vi "Main.vi"() -> ()   [LabVIEW 2017]
uses:
  type defs/action buttons.ctl
  type defs/mode buttons.ctl
  <vilib>/vision/Pattern Matching.llb/IMAQ GM Match Report.ctl
  type defs/states.ctl
  type defs/data.ctl
  <vilib>/vision/Image Controls.llb/IMAQ Image.ctl
  <vilib>/myRIO/Common/Instrument Driver Framework/myRIO v1.0/Encoder/typedefs/Encoder Signal Mode.ctl
  <vilib>/myRIO/Instrument Drivers/Onboard IO/PWM/typedefs/PWM Reference.ctl
  <vilib>/myRIO/Common/Instrument Driver Framework/Utilities/typedefs/myRIO Generic Hardware Reference.ctl
  <vilib>/myRIO/Common/Instrument Driver Framework/Utilities/typedefs/Hardware Version Enum.ctl
  <vilib>/myRIO/Common/Instrument Driver Framework/Utilities/typedefs/myRIO v1.0 Reference.ctl
  <vilib>/myRIO/Common/Instrument Driver Framework/Utilities/typedefs/Generic FPGA Reference.ctl
  <vilib>/myRIO/Common/Instrument Driver Framework/myRIO v1.0/PWM/typedefs/PWM Channels Enum.ctl
  <vilib>/myRIO/Instrument Drivers/Onboard IO/PWM/typedefs/PWM Configuration.ctl
  <vilib>/userdefined/High Color/nirio_resource_hc.ctl
  <vilib>/myRIO/Instrument Drivers/Onboard IO/DIO/typedefs/DIO Reference.ctl
  <vilib>/myRIO/Common/Instrument Driver Framework/myRIO v1.0/DIO/typedefs/DIO Channels List.ctl
  <vilib>/myRIO/Common/Instrument Driver Framework/myRIO v1.0/DIO/typedefs/DIO Channels Enum.ctl
  type defs/task.ctl
  <vilib>/myRIO/Common/Instrument Driver Framework/Utilities/vis/Is FPGA Ref Available.vi
  <vilib>/myRIO/Common/Instrument Driver Framework/myRIO v1.0/PWM/vis/myRIO v1.1 Open PWM.vi
  <vilib>/myRIO/Common/Instrument Driver Framework/myRIO v1.0/DIO/vis/myRIO v1.1 Open DIO.vi
  <vilib>/myRIO/Instrument Drivers/Onboard IO/DIO/vis/Write.vi
  <vilib>/myRIO/Common/Instrument Driver Framework/Utilities/vis/Validate Channels.vi
  <vilib>/myRIO/Common/Instrument Driver Framework/myRIO v1.0/PWM/vis/myRIO v1.0 Reserve PWM.vi
  <vilib>/myRIO/Common/Instrument Driver Framework/myRIO v1.0/DIO/vis/myRIO v1.0 Reserve DIO.vi
  <vilib>/myRIO/Common/Instrument Driver Framework/myRIO v1.0/Encoder/vis/myRIO v1.0 Close Encoder.vi
  <vilib>/myRIO/Common/Instrument Driver Framework/myRIO v1.0/PWM/vis/myRIO v1.0 Close PWM.vi
  <vilib>/myRIO/Common/Instrument Driver Framework/myRIO v1.0/UART/vis/myRIO v1.0 Close UART.vi
  <vilib>/myRIO/Common/Instrument Driver Framework/myRIO v1.0/PWM/vis/myRIO v1.0 Build MUX Configuration PWM.vi
  <vilib>/myRIO/Common/Instrument Driver Framework/myRIO v1.0/Resource Manager/vis/myRIO v1.0 Reserve Channel List.vi
  <vilib>/myRIO/Common/Instrument Driver Framework/myRIO v1.0/DIO/vis/myRIO v1.0 Build MUX Configuration DIO.vi
  <vilib>/myRIO/Common/Instrument Driver Framework/myRIO v1.0/Encoder/vis/myRIO v1.0 Unreserve Encoder.vi
  <vilib>/myRIO/Common/Instrument Driver Framework/myRIO v1.0/PWM/vis/myRIO v1.0 Unreserve PWM.vi
  <vilib>/myRIO/Common/Instrument Driver Framework/myRIO v1.0/Resource Manager/vis/myRIO v1.0 Create Configuration List.vi
  <vilib>/myRIO/Common/Instrument Driver Framework/myRIO v1.0/Resource Manager/vis/myRIO v1.0 Reserve Channel.vi
  <vilib>/myRIO/Common/Instrument Driver Framework/myRIO v1.0/Resource Manager/vis/myRIO v1.0 Unreserve Channel.vi
  <vilib>/myRIO/Common/Instrument Driver Framework/myRIO v1.0/Encoder/vis/myRIO v1.0 Build MUX Configuration Encoder.vi
  <vilib>/myRIO/Common/Instrument Driver Framework/myRIO v1.0/Resource Manager/vis/myRIO v1.0 Unreserve Channel List.vi
  <vilib>/myRIO/Common/Instrument Driver Framework/myRIO v1.0/Resource Manager/vis/myRIO v1.0 Build Mutex Name.vi
  <vilib>/Utility/VariantDataType/GetNumericInfo.vi
  <vilib>/Utility/error.llb/Error Cluster From Error Code.vi
  <vilib>/myRIO/Common/Instrument Driver Framework/myRIO v1.0/myRIO v1.1 Open.vi
  <vilib>/myRIO/Common/Instrument Driver Framework/Utilities/vis/IO Manager.vi
  <vilib>/myRIO/Common/Instrument Driver Framework/Utilities/vis/Configuration Manager.vi
  <vilib>/myRIO/Common/Instrument Driver Framework/myRIO v1.0/Resource Manager/vis/myRIO v1.0 Configure IO.vi
  <vilib>/myRIO/Common/Instrument Driver Framework/myRIO v1.0/myRIO v1.0 Close.vi
  <vilib>/myRIO/Common/Instrument Driver Framework/myRIO v1.0/Encoder/vis/myRIO v1.0 Reset Encoder.vi
  <vilib>/myRIO/Common/Instrument Driver Framework/myRIO v1.0/PWM/vis/myRIO v1.0 Write PWM.vi
  <vilib>/myRIO/Common/Instrument Driver Framework/myRIO v1.0/Encoder/vis/myRIO v1.0 Read Encoder.vi
  <vilib>/myRIO/Common/Instrument Driver Framework/myRIO v1.0/DIO/vis/myRIO v1.0 Write DIO.vi
  <vilib>/myRIO/Common/Instrument Driver Framework/myRIO v1.0/DIO/vis/myRIO v1.0 Read DIO.vi
  <vilib>/myRIO/Common/Instrument Driver Framework/myRIO v1.0/PWM/vis/myRIO v1.0 Shutdown PWM.vi
  <vilib>/myRIO/Common/Instrument Driver Framework/myRIO v1.0/Encoder/vis/myRIO v1.0 Shutdown Encoder.vi
  <vilib>/myRIO/Common/Instrument Driver Framework/Utilities/vis/FPGA Ref Manager.vi
  <vilib>/myRIO/Common/Instrument Driver Framework/myRIO v1.0/myRIO v1.0 Reset FPGA.vi
  <vilib>/myRIO/Common/Instrument Driver Framework/myRIO v1.0/IRQ/vis/myRIO v1.0 IRQ Info FGV.vi
  <vilib>/myRIO/Common/Instrument Driver Framework/myRIO v1.0/IRQ/vis/myRIO v1.0 Timer IRQ Info FGV.vi
  <vilib>/myRIO/Common/Instrument Driver Framework/myRIO v1.0/IRQ/vis/myRIO v1.0 ISR Agent.vi
  <vilib>/myRIO/Instrument Drivers/Onboard IO/I2C/typedefs/I2C Reference.ctl
  <vilib>/myRIO/Common/Instrument Driver Framework/myRIO v1.0/I2C/typedefs/I2C Channels Enum.ctl
  <vilib>/myRIO/Instrument Drivers/Onboard IO/I2C/typedefs/I2C Configuration.ctl
  <vilib>/myRIO/Instrument Drivers/Onboard IO/I2C/typedefs/I2C Transfer Rate.ctl
  <vilib>/myRIO/Express VI/Onboard IO/PWM/PWM Express VI.xnode
  <vilib>/myRIO/Instrument Drivers/Onboard IO/PWM/vis/myRIO PWM Open.xnode
  <vilib>/myRIO/Express VI/Onboard IO/DO/DO Express VI.xnode
  <vilib>/myRIO/Instrument Drivers/Onboard IO/DIO/vis/myRIO DIO Open.xnode
  <vilib>/myRIO/Express VI/Onboard Devices/LED/LED Express VI.xnode
  <vilib>/myRIO/Express VI/Onboard Devices/Button/Button Express VI.xnode
  <vilib>/myRIO/Instrument Drivers/Onboard IO/DIO/DIO.lvlib
  <vilib>/myRIO/Instrument Drivers/Onboard IO/PWM/PWM.lvlib
  <vilib>/myRIO/Instrument Drivers/Utilities/Utilities.lvlib
  <vilib>/vision/NI_Vision_Development_Module.lvlib
  <vilib>/myRIO/Instrument Drivers/Onboard IO/I2C/I2C.lvlib
  <vilib>/myRIO/Instrument Drivers/Onboard IO/I2C/vis/myRIO I2C Open.xnode
  <vilib>/myRIO/Common/Instrument Driver Framework/myRIO v1.0/I2C/vis/myRIO v1.1 Open I2C.vi
  <vilib>/myRIO/Instrument Drivers/Onboard IO/Encoder/Encoder.lvlib
panel:
  in  "Def PWM":dbl=0.5
  out "CurState":T1(ring)
  out "Found Right Ball":bool=TRUE
  out "FT_G_enc":i32[](array[numeric])
  out "FT_M_enc":i32[](array[numeric])
  out "FT_Right_enc":i32[](array[numeric])
  out "FT_Left_enc":i32[](array[numeric])
  out "FT_Angles":dbl[](array[numeric])
  out "Dots of States":i32[][](array[numeric])
  in  "States in total":i32
  in  "(auto) States":T2(ring)
  out "G_enc":i32[](array[numeric])
  out "M_enc":i32[](array[numeric])
  out "Right_enc":i32[](array[numeric])
  out "Left_enc":i32[](array[numeric])
  out "Angles":dbl[](array[numeric])
  in  "Dots in total":i32
  in  "CurDot":T3(ring)
  out "(auto) balls counter":i32
  out "distance to the side":u32
  out "value Z 2":ext
  out "value Z":ext
  in  ",ctl num":i32
  in  ".Task":enum16{"Def", "<mod>[P]+tnl ", "(auto)"}(ring)
  out "Pattern classes":i32[](array[numeric])
  in  "5":i32
  in  "4":i32
  in  "3":i32
  in  "1":i32
  in  "2":i32
  out "5b":bool
  out "4b":bool
  out "3b":bool
  out "2b":bool
  out "1b":bool
  out "Color classes":i32[](array[numeric])
  in  "Next step":bool
  in  "ball = pattern?":bool
  out "error out":errorcluster
  in  "Tab Control":enum32{"Motors", "Ball", "Pattern", "Camera"}(tab)
  in  "Left+":bool
  in  "Left-":bool
  in  "Right+":bool
  in  "Right-":bool
  in  "G-":bool
  in  "G+":bool
  in  "M+":bool
  in  "M-":bool
  in  "M_PWM":dbl=0.5
  in  "L_PWM":dbl=0.5
  in  "R_PWM":dbl=0.5
  in  "Reset M_enc":bool
  out "M_enc_value":i32
  in  "Reset G_enc":bool
  out "G_enc_value":i32
  in  "G_PWM":dbl=0.5
  in  "M_UB_Align":i32=-800
  in  "G_UB_Align":i32
  in  "M_UB_grab":i32=-800
  in  "G_UB_grab":i32=-500
  in  "Manip state":enum16{"Align", "Grab", "Release"}(ring)
  in  "Reset L_enc":bool
  out "L_enc_value":i32
  in  "Reset R_enc":bool
  out "R_enc_value":i32
  in  "Balls to remember":i32
  out "Circles Calibrated (Shape Detection 1)":T4(array[cluster]) {"Position"."Y" format="%.2f"; "Position"."X" format="%.2f"}
  out "Number of Matches (Shape Detection 1)":i32
  out "Color":i32
  in  "Align X - t, Y - f":bool
  out "CircleRadius":dbl
  in  "defX":dbl=360.0
  in  "RangeY":dbl=30.0
  in  "defY":dbl=380.0
  out "X is in range":bool
  out "Y is in range":bool
  out "curX":dbl
  out "curY":dbl
  out "1y1 (circle)":i32
  out "1x1 (circle)":i32
  out "1x0 (circle)":i32
  out "1y0 (circle)":i32
  in  "divider (circle)":dbl=1.0
  in  "ROI Descriptor COLOR":T5={"Global Rectangle"=[86, 71, 180, 164], "Contours"=[{"ID"=enum."External", "Type"=3, "Coordinates"=[86, 71, 180, 164]}]} {"Contours"."Type" items=["No Selection", "Point", "Line", "Rectangle", "Oval", "Polygon", "Freehand Region", "Annulus", "Unused2", "Unused3", "Broken Line", "Freehand Line", "Rotated Rectangle"]}
  in  "align accuracy":u32=100
  in  "Ball number":i32=1
  out "ball match":bool
  in  "RangeX":dbl=40.0
  out "Ready to Grab":bool
  in  "Range(p)":sgl=10.0
  in  "defX(p)":sgl=320.0
  out "Pattern":i32
  out "y0":i32
  out "x0":i32
  out "x1":i32
  out "y1":i32
  out "Number of Matches (Geometric Matching 1)":i32
  out "Calibrated Matches (Geometric Matching 1)":T6[](array[typedef]) {"Correlation Score" format="%.2f"; "Target Template Curve Score" format="%.2f"; "Template Target Curve Score" format="%.2f"; "Bounding Box"."y" format="%.2f"; "Bounding Box"."x" format="%.2f"; "Position"."y" format="%.2f"; "Position"."x" format="%.2f"; "Score" format="%.2f"; "Scale" format="%.2f"; "Angle" format="%.2f"; "Occlusion %" format="%.2f"}
  out "Scale":sgl
  in  "divider (pattern)":sgl=1.0
  out "curX(p)":sgl
  out "In Range? (p)":bool
  in  "align accuracy (p)":u32=100
  in  "pattern number":i32=1
  in  "patterns to remember":i32=3
  out "pattern match":bool
  in  "M duty cycle [P]":dbl=533.0 format="%#_13g"
  in  "S duty cycle [P]":dbl=990.0 format="%#_13g"
  in  "S duty cycle [B]":dbl=990.0 format="%#_13g"
  in  "M duty cycle [B]":dbl=533.0 format="%#_13g"
  in  "S duty cycle [F]":dbl=620.0 format="%#_13g"
  in  "M duty cycle [F]":dbl=506.0 format="%#_13g"
  in  "Angle for pattern (degrees)":sgl=90.0 format="%.2f"
  out "rotate":bool=TRUE
  in  "PWM channel (m)":tag="B/PWM2"
  in  "[cur] duty cycle [%] (m)":dbl
  in  "PWM channel (s)":tag="A/PWM2"
  in  "[cur] duty cycle [%] (s)":dbl
  in  "Camera state":enum16{"Fwd", "Pattern", "Ball"}(ring)
  in  "Angle for Align (degrees)":sgl=2.0 format="%.2f"
  in  "mode buttons":T7
  out "image display":T8(plugin-control)
  in  "action buttons":T9
  in  "Stop":bool
  # "Machine\nVision\nApp"
  # "less = slower"
  # "less = slower"
  # "0 - 640x480"
  # "5 - 1280x720"
  # "30 - 320x240"
  # "35 - 800x600"
  # "40 - 176x144"
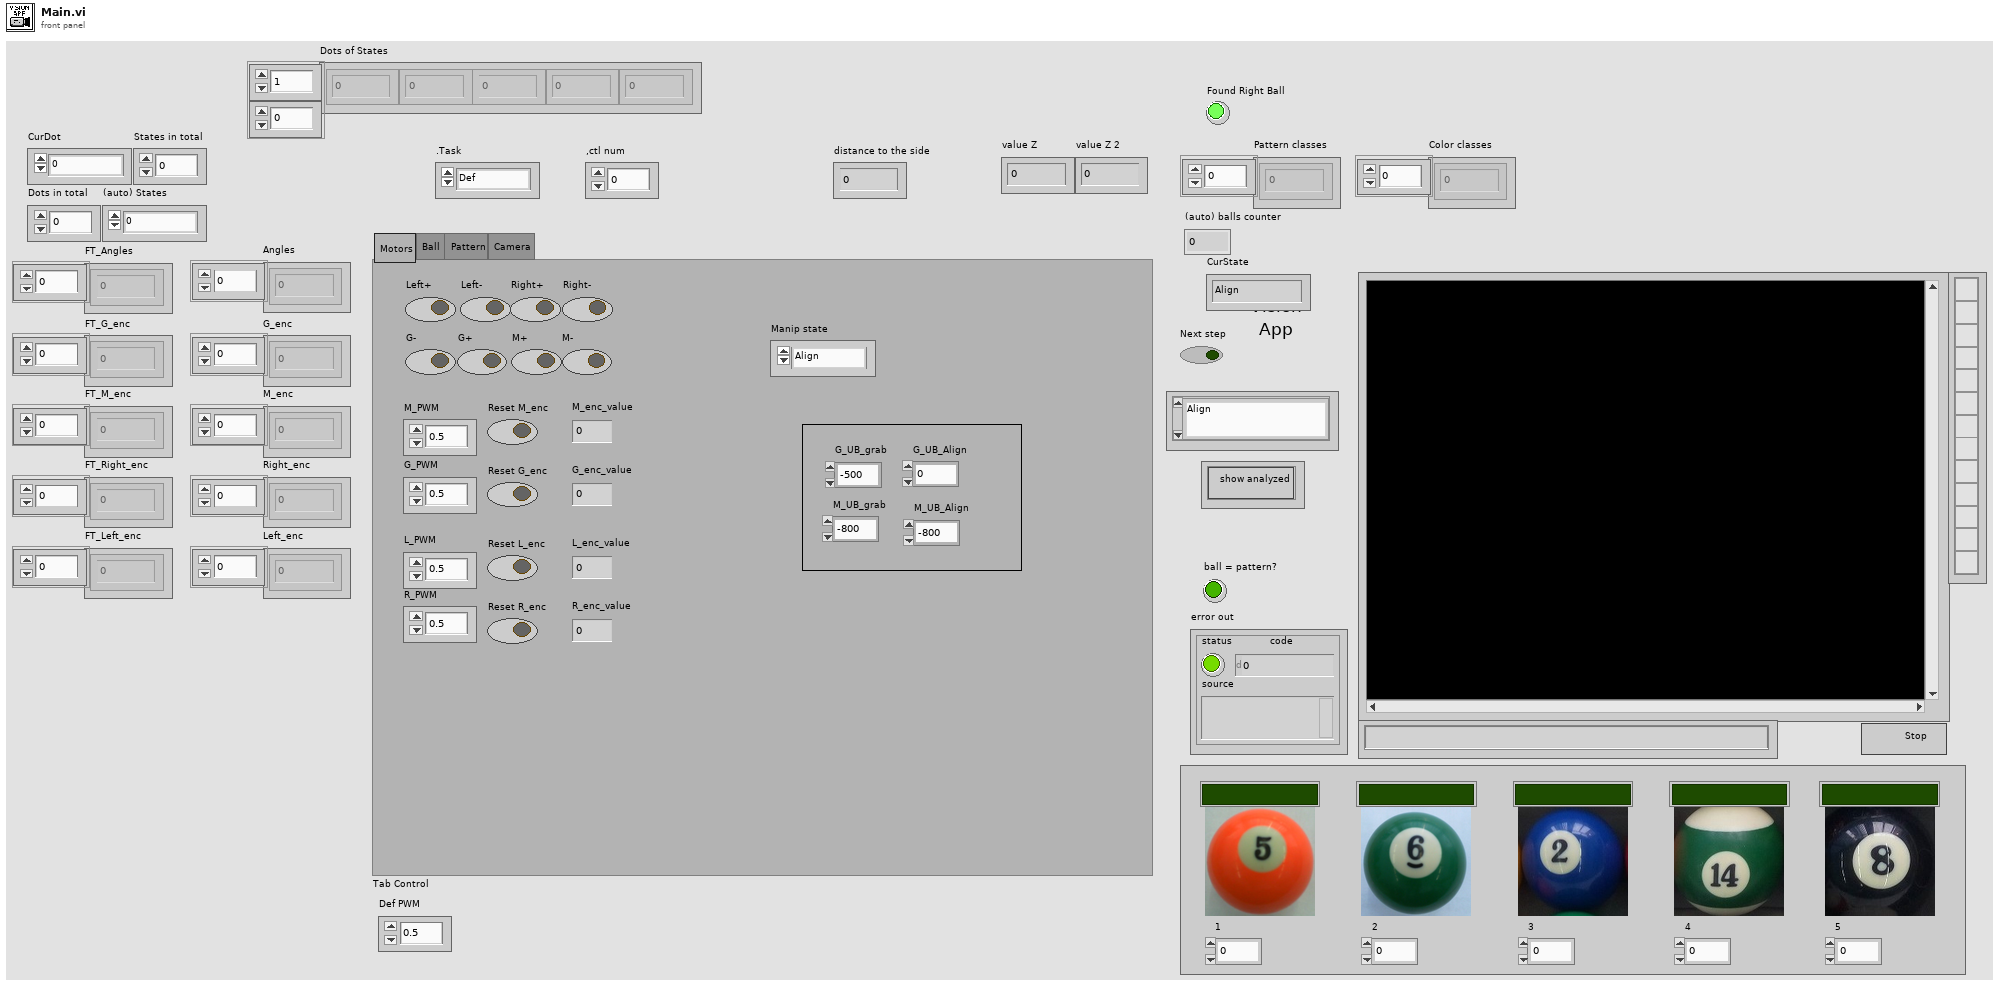
[diagram p1: front panel]
types:
  T1 = enum16{"Align", "1", "2", "3", "4", "5", "6", "7", "8", "9", "10", "11", "12", "13", "(pattern) Align", "Pattern", "(mod) pattern", "<mod>[P] remembering", "<mod>[P] go through tunnel", "<mod>[P] comparing", "(mod) ball", "Ball", "Other", "Clear", "navx", "(auto) Balls Analyze", "(auto) Ball Analyze", "(pattern) Align <loop>", "(ball) Align <loop>", "Joystick control"}
  T2 = enum16{"0", "1", "2", "3", "4", "5", "6", "7", "8", "9", "10"}
  T3 = enum16{"0", "1", "2", "3", "4", "5", "6", "7", "8", "9", "10", "11", "12", "13", "14", "15", "16", "17", "18", "19", "20", "21", "22", "23", "24", "25", "26", "27", "28", "29", "30", "31", "32", "33", "34", "35"}
  T4 = cluster{"Position":cluster{"X":sgl, "Y":sgl}, "Radius":dbl, "Score":dbl}[]
  T5 = cluster{"Global Rectangle":i32[], "Contours":cluster{"ID":enum32{"External", "Internal"}, "Type":u32, "Coordinates":i32[]}[]}
  T6 = typedef "IMAQ GM Match Report.ctl" = cluster{"Position":cluster{"x":sgl, "y":sgl}, "Angle":sgl, "Scale":sgl, "Score":sgl, "Bounding Box":cluster{"x":sgl, "y":sgl}[], "Contrast Reversed":bool, "Occlusion %":sgl, "Template Target Curve Score":sgl, "Target Template Curve Score":sgl, "Correlation Score":sgl}
  T7 = typedef "mode buttons.ctl" = cluster{"show analyzed":bool}
  T8 = typedef "IMAQ Image.ctl" = refnum<image>
  T9 = typedef "action buttons.ctl" = cluster{"State":enum16{"Align", "1", "2", "3", "4", "5", "6", "7", "8", "9", "10", "11", "12", "13", "(pattern) Align", "Pattern", "(mod) pattern", "<mod>[P] remembering", "<mod>[P] go through tunnel", "<mod>[P] comparing", "(mod) ball", "Ball", "Other", "Clear", "navx", "(auto) Balls Analyze", "(auto) Ball Analyze", "(pattern) Align <loop>", "(ball) Align <loop>", "Joystick control"}}
  T10 = typedef "Encoder Signal Mode.ctl" = enum16{"Quadrature phase signal", "Step and direction signal"}
  T11 = typedef "data.ctl" = cluster{"Shape - t, Color - f":bool, "qsm":cluster{"Webcam image ref":T8, "Analyzed image ref":T8, "Stop webcam":bool}, " image ref":T8, "number img":i32, "ROI Descriptor (Image Mask 1)":cluster{"Global Rectangle":i32[], "Contours":cluster{"ID":enum32{"External", "Internal"}, "Type":u32, "Coordinates":i32[]}[]}, "Pattern class":i32, "Color class":i32, "Color classes":i32[], "Pattern classes":i32[]}
  T12 = typedef "states.ctl" = enum16{"(qsm) schedule", "(qsm) initialize", "(qsm) release", "(qsm) clean up", "(qsm) shutdown", "(myRIO) initialize", "(myRIO) clean up", "(myRIO) update ports", "Setup get", "(image) get", "(image) show", "(ball) Shape detection", "(ball) Calc ball indx", "(ball) Calculate ROI", "(ball) Analyze color", "(ball) Align", "(ball) Wait", "(ball) Grab", "(pattern) Find Square", "(pattern) Calculate ROI", "(pattern) Calc pattern indx", "Compare", "(pattern) Analyze pattern", "(pattern) Align", "(pattern) Wait", "(pattern) states control", "navx", "stop motors", "(joystick) Joystick control", "_Timer", "Setup manipulator", "(auto) Count balls", "(auto) Analyze balls", "(auto) Dot Controller", "(auto) Fwd (cm)", "(auto) Turn (angle)", "(auto) Tnl (M2-M2.5)", "Wait for button"}
  T13 = typedef "Encoder.lvlib/Encoder Reference.ctl" = cluster{"myRIO Reference":T14, "Encoder Channels Enum":T18}
  T14 = typedef "myRIO Generic Hardware Reference.ctl" = cluster{"myRIO Model":T15, "myRIO Hardware Reference":T16}
  T15 = typedef "Hardware Version Enum.ctl" = enum16{"Unknown", "myRIO-1900", "myRIO-1950", "roboRIO", "NI ELVIS RIO CM"}
  T16 = typedef "myRIO v1.0 Reference.ctl" = cluster{"Generic FPGA Reference":T17, "Allow multiple opens":bool}
  T17 = typedef "Generic FPGA Reference.ctl" = refnum<k20>
  T18 = typedef "Encoder Channels Enum.ctl" = enum16{"Not Connected", "C/ENC0", "C/ENC1", "A/ENC", "B/ENC", "DIO/ENC0", "DIO/ENC1", "DIO/ENC2", "DIO/ENC3", "DIO/ENC4"}
  T19 = typedef "PWM.lvlib/PWM Reference.ctl" = cluster{"myRIO Reference":T14, "PWM Channels Enum":T20, "PWM Configuration":T21}
  T20 = typedef "PWM Channels Enum.ctl" = enum16{"Not Connected", "C/PWM0", "C/PWM1", "A/PWM0", "A/PWM1", "A/PWM2", "B/PWM0", "B/PWM1", "B/PWM2", "PWM/PWM0", "PWM/PWM1", "PWM/PWM2", "PWM/PWM3", "PWM/PWM4", "PWM/PWM5", "PWM/PWM6", "PWM/PWM7", "PWM/PWM8", "PWM/PWM9"}
  T21 = typedef "PWM.lvlib/PWM Configuration.ctl" = cluster{"Frequency":dbl, "Duty Cycle":dbl}
  T22 = typedef "nirio_resource_hc.ctl" = tag
  T23 = typedef "I2C.lvlib/I2C Reference.ctl" = cluster{"myRIO Reference":T14, "I2C Channels Enum":T24, "I2C Configuration":T25}
  T24 = typedef "I2C Channels Enum.ctl" = enum16{"Not Connected", "A/I2C", "B/I2C", "I2C/I2C"}
  T25 = typedef "I2C.lvlib/I2C Configuration.ctl" = cluster{"I2C Transfer Rate":T26}
  T26 = typedef "I2C.lvlib/I2C Transfer Rate.ctl" = enum16{"Standard mode (100 kbps)", "Fast mode (400 kbps)"}
  T27 = typedef "DIO.lvlib/DIO Reference.ctl" = cluster{"myRIO Reference":T14, "DIO Channels List":T28}
  T28 = typedef "DIO Channels List.ctl" = T29[]
  T29 = typedef "DIO Channels Enum.ctl" = enum16{"Not Connected", "C/DIO0", "C/DIO1", "C/DIO2", "C/DIO3", "C/DIO4", "C/DIO5", "C/DIO6", "C/DIO7", "A/DIO0", "A/DIO1", "A/DIO2", "A/DIO3", "A/DIO4", "A/DIO5", "A/DIO6", "A/DIO7", "A/DIO8", "A/DIO9", "A/DIO10", "A/DIO11", "A/DIO12", "A/DIO13", "A/DIO14", "A/DIO15", "B/DIO0", "B/DIO1", "B/DIO2", "B/DIO3", "B/DIO4", "B/DIO5", "B/DIO6", "B/DIO7", "B/DIO8", "B/DIO9", "B/DIO10", "B/DIO11", "B/DIO12", "B/DIO13", "B/DIO14", "B/DIO15", "LED0", "LED1", "LED2", "LED3", "Button0", "DIO/DIO0", "DIO/DIO1", "DIO/DIO2", "DIO/DIO3", "DIO/DIO4", "DIO/DIO5", "DIO/DIO6", "DIO/DIO7", "DIO/DIO8", "DIO/DIO9", "SPI/CS0", "SPI/CS1", "SPI/CS2", "SPI/CS3", "LED RADIO (Green)", "LED RADIO (Red)", "LED COMM (Green)", "LED COMM (Red)", "LED MODE (Green)", "LED MODE (Red)"}
  T30 = enum16{"Align", "(pattern) Align", "Pattern", "(mod) pattern", "(mod) ball", "Ball", "Other", "Clear", "Joystick control"}
  T31 = enum16{"Align", "(pattern) Align", "Pattern", "(mod) pattern", "<mod>[P] remembering", "<mod>[P] go through tunnel", "<mod>[P] comparing", "(mod) ball", "Ball", "Other", "Clear", "Joystick control"}
  T32 = enum16{"Align", "(pattern) Align", "Pattern", "(mod) pattern", "<mod>[P]+move", "(mod) ball", "Ball", "Other", "Clear", "Joystick control"}
  T33 = typedef "task.ctl" = T12[]
  T34 = typedef "Image Type" = u32
  T35 = cluster{"Position":cluster{"X":sgl, "Y":sgl}, "Radius":dbl, "Score":dbl}
  T36 = cluster{"ID":enum32{"External", "Internal"}, "Type":u32, "Coordinates":i32[]}[]
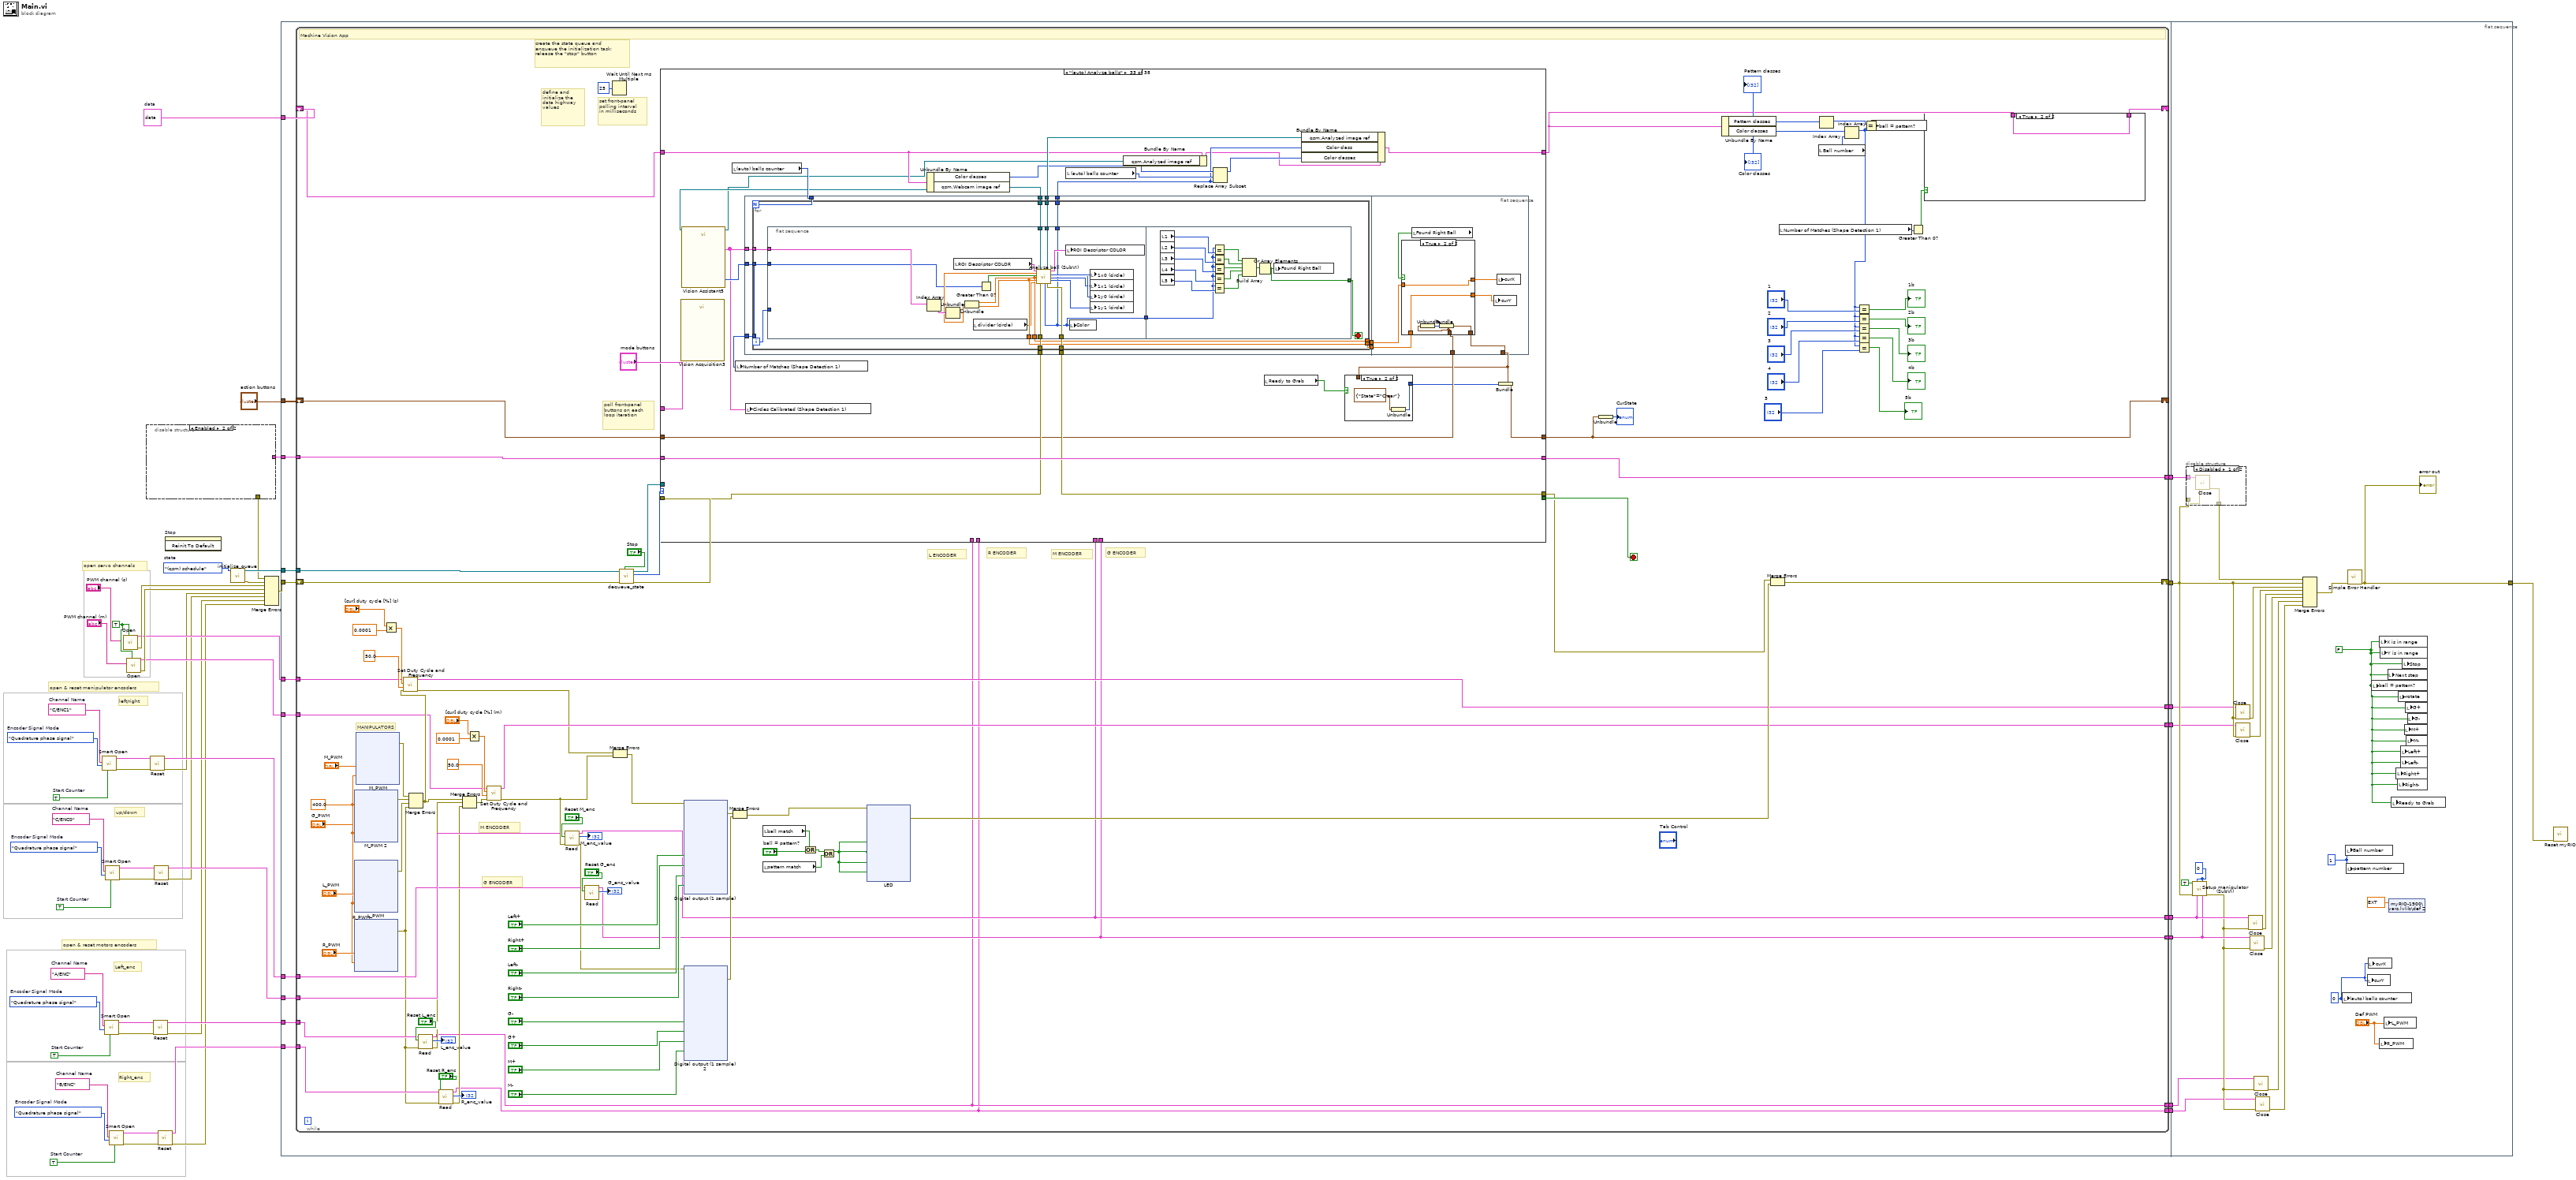
[diagram p0: block diagram]
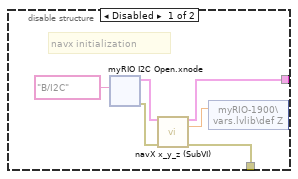
[diagram p2: hidden frame]
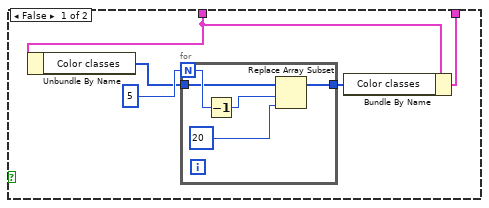
[diagram p3: hidden frame]
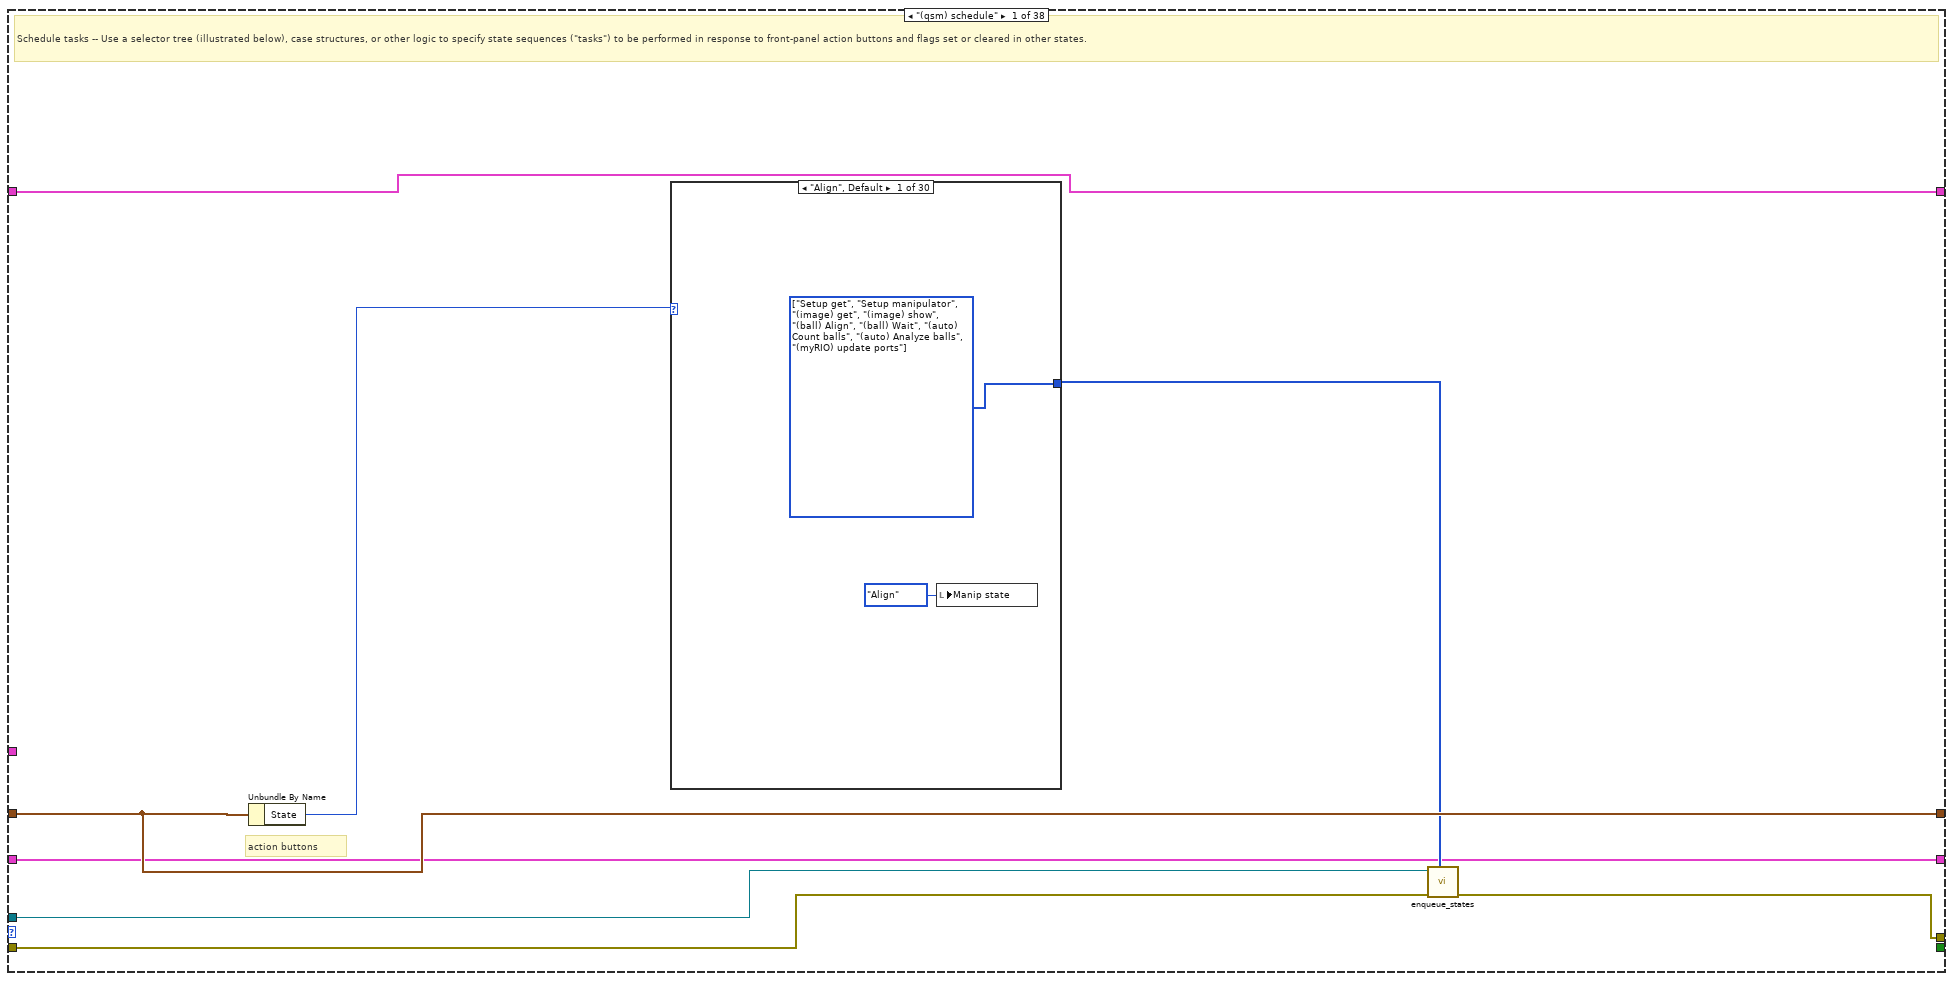
[diagram p4: hidden frame]
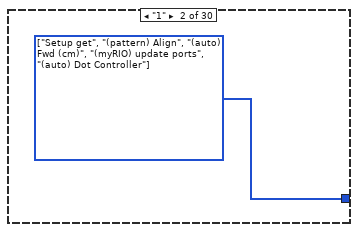
[diagram p5: hidden frame]
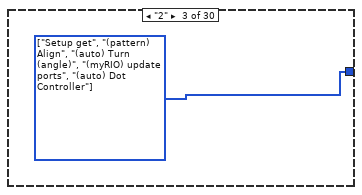
[diagram p6: hidden frame]
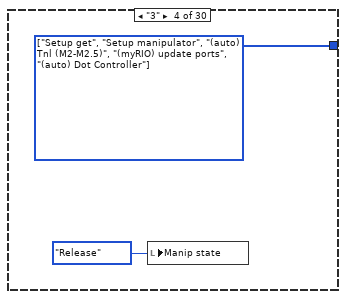
[diagram p7: hidden frame]
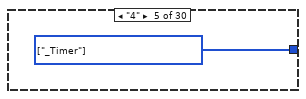
[diagram p8: hidden frame]
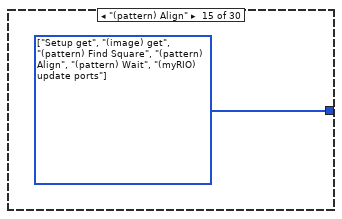
[diagram p18: hidden frame]
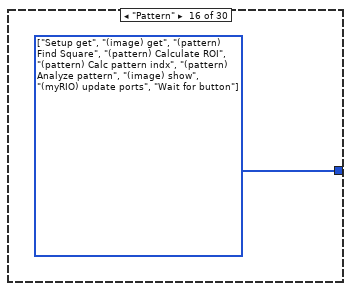
[diagram p19: hidden frame]
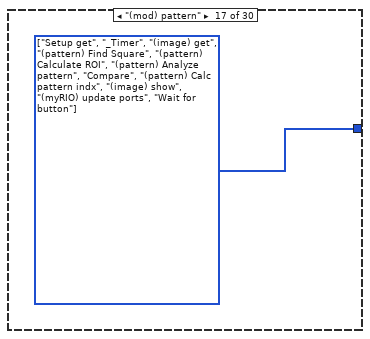
[diagram p20: hidden frame]
diagram:
  w8 = TRUE  # Start Counter
  w7 = TRUE  # Start Counter
  w11 = Encoder_Signal_Mode."Quadrature phase signal"  # Encoder Signal Mode
  w12 = tag "B/ENC"  # Channel Name
  w15 = Encoder_Signal_Mode."Quadrature phase signal"  # Encoder Signal Mode
  w16 = tag "A/ENC"  # Channel Name
  w24 = TRUE  # Start Counter
  w25 = Encoder_Signal_Mode."Quadrature phase signal"  # Encoder Signal Mode
  w26 = tag "C/ENC1"  # Channel Name
  w30 = TRUE  # Start Counter
  w31 = Encoder_Signal_Mode."Quadrature phase signal"  # Encoder Signal Mode
  w32 = tag "C/ENC0"  # Channel Name
  w39 = TRUE ("Allow multiple opens?")
  w36 = T11 {"Shape - t, Color - f"=FALSE, "qsm"={"Webcam image ref"=refnum, "Analyzed image ref"=refnum, "Stop webcam"=FALSE}, " image ref"=refnum, "number img"=0, "ROI Descriptor (Image Mask 1)"={"Global Rectangle"=[109, 72, 345, 284], "Contours"=[{"ID"=enum."External", "Type"=3, "Coordinates"=[109, 72, 345, 284]}]}, "Pattern class"=0, "Color class"=0, "Color classes"=[], "Pattern classes"=[]}  # data
  w47 = states."(qsm) schedule"  # state
  # "open & reset motors encoders"
  # "Right_enc"
  # "Left_enc"
  # "left/right"
  # "up/down"
  # "open servo channels"
  # "open & reset manipulator encoders"
  n1 = call <vilib>:"Smart Open.vi"("Start Counter"=w24, "Encoder Signal Mode"=w25, "Channel Name"=w26) -> ("error out"=w22:errorcluster, "Encoder Ref Out"=w23:T13)  [unwired: 7 in]
  n2 = call <vilib>:"Smart Open.vi"("Start Counter"=w7, "Encoder Signal Mode"=w15, "Channel Name"=w16) -> ("error out"=w13:errorcluster, "Encoder Ref Out"=w14:T13)  [unwired: 7 in]
  n3 = call <vilib>:"Smart Open.vi"("Start Counter"=w30, "Encoder Signal Mode"=w31, "Channel Name"=w32) -> ("error out"=w28:errorcluster, "Encoder Ref Out"=w29:T13)  [unwired: 7 in]
  n4 = call <vilib>:"Smart Open.vi"("Start Counter"=w8, "Encoder Signal Mode"=w11, "Channel Name"=w12) -> ("error out"=w9:errorcluster, "Encoder Ref Out"=w10:T13)  [unwired: 7 in]
  n5 = call <vilib>:"Open.vi"("Allow multiple opens?"=w39, "Channel Name"="PWM channel (s)") -> ("error out"=w45:errorcluster, "PWM Ref Out"=w43:T19)  [unwired: 8 in]
  n6 = call <vilib>:"Open.vi"("Allow multiple opens?"=w39, "Channel Name"="PWM channel (m)") -> ("error out"=w44:errorcluster, "PWM Ref Out"=w42:T19)  [unwired: 8 in]
  n7 = disable-structure shown="Enabled" {
    disable-tunnel: [w56 _] -> w34
    disable-tunnel: [w54 _] -> w33
    frame Disabled {
      # "navx initialization"
      n8 = xnode "myRIO I2C Open.xnode"("Channel Name"=tag "B/I2C") -> ("error out"=w53:errorcluster, "I2C Ref Out"=w55:T23)  [unwired: 2 in]
      n9 = call "navX x_y_z (SubVI).vi"("I2C Ref Out in"=w55, "error in (no error)"=w53) -> ("I2C Ref Out out"=w54:T23, "value Z"=w57:ext, "error out"=w56:errorcluster)  [unwired: 9 in, 2 out]
      n10 = shared-variable "myRIO-1900\\vars.lvlib\\def Z"(w57) -> ()  [unwired: 1 in, 1 out]
    }
    frame Enabled {
    }
  }
  n11 = call <vilib>:"Reset.vi"("error in (no error)"=w22, "Encoder Ref In"=w23) -> ("error out"=w17:errorcluster, "Encoder Ref Out"=w21:T13)  [unwired: 8 in]
  n12 = call <vilib>:"Reset.vi"("error in (no error)"=w13, "Encoder Ref In"=w14) -> ("error out"=w4:errorcluster, "Encoder Ref Out"=w6:T13)  [unwired: 8 in]
  n13 = call <vilib>:"Reset.vi"("error in (no error)"=w28, "Encoder Ref In"=w29) -> ("error out"=w18:errorcluster, "Encoder Ref Out"=w27:T13)  [unwired: 8 in]
  n14 = call <vilib>:"Reset.vi"("error in (no error)"=w9, "Encoder Ref In"=w10) -> ("error out"=w3:errorcluster, "Encoder Ref Out"=w5:T13)  [unwired: 8 in]
  n15 = invoke on="Stop" class="Bool (strict)" method="Reinit To Default"() -> ()  [unwired: 3 in, 3 out]
  n16 = call "initialize_queue.vi"("state"=w47) -> ("error out"=w48:errorcluster, "queue out"=w49:refnum<queue>)  [unwired: 9 in]
  n17 = Merge Errors(w34, w48, w45, w44, w17, w18, w4, w3) -> (w46:errorcluster)
  n18 = flat-sequence {
    tunnel: [w93] -> w51
    tunnel: "action buttons" -> [w92]
    tunnel: w46 -> [w90]
    tunnel: w49 -> [w91]
    tunnel: w36 -> [w89]
    tunnel: w43 -> [w88]
    tunnel: w42 -> [w87]
    tunnel: [w86] -> w41
    tunnel: [w85] -> w40
    tunnel: w33 -> [w84]
    tunnel: [w83] -> w35
    tunnel: w27 -> [w82]
    tunnel: w21 -> [w81]
    tunnel: [w80] -> w20
    tunnel: [w79] -> w19
    tunnel: w6 -> [w78]
    tunnel: w5 -> [w77]
    tunnel: [w76] -> w2
    tunnel: [w75] -> w1
    tunnel: [w1391] -> w52
    tunnel: w51 -> [w1381]
    tunnel: w41 -> [w1379]
    tunnel: w40 -> [w1378]
    tunnel: w35 -> [w1386]
    tunnel: w20 -> [w1376]
    tunnel: w19 -> [w1377]
    tunnel: w2 -> [w1372]
    tunnel: w1 -> [w1373]
    frame #0 {
      n19 = while {
        shift-right: [w186] -> w93
        shift-left: w90 -> [w191]
        shift-right: [w167] -> _
        shift-left: w89 -> [w94]
        shift-right: [w97] -> _
        shift-left: w92 -> [w175]
        tunnel: w91 -> [w174]
        tunnel: w88 -> [w136]
        tunnel: w87 -> [w120]
        tunnel: [w133] -> w86
        tunnel: [w132] -> w85
        tunnel: w84 -> [w130]
        tunnel: [w129] -> w83
        tunnel: w82 -> [w122]
        tunnel: w81 -> [w121]
        tunnel: [w118] -> w80
        tunnel: [w119] -> w79
        tunnel: w78 -> [w105]
        tunnel: w77 -> [w104]
        tunnel: [w99] -> w76
        tunnel: [w98] -> w75
        stop <- w173 stop-if-true
        w111 = 400.0 ("Frequency [Hz]")
        # "R ENCODER"
        # "L ENCODER"
        # "G ENCODER"
        # "M ENCODER"
        # "G ENCODER"
        # "M ENCODER"
        # "define and \ninitialize the \ndata highway\nvalues"
        # "MANIPULATORS"
        # "create the state queue and\nenqueue the initialization task;\nrelease the \"stop\" button"
        # "set front-panel\npolling interval\nin milliseconds"
        # "poll front-panel\nbuttons on each\nloop iteration"
        # "Machine Vision App"
        n20 = xnode "M_PWM 2"("Duty Cycle"="G_PWM", "Frequency [Hz]"=w111) -> ("error out"=w112:errorcluster)  [unwired: 1 in]
        n21 = xnode "L_PWM"("Duty Cycle"="L_PWM", "Frequency [Hz]"=w111) -> ("error out"=w185:errorcluster)  [unwired: 1 in]
        n22 = xnode "R_PWM"("Duty Cycle"="R_PWM", "Frequency [Hz]"=w111) -> ("error out"=w103:errorcluster)  [unwired: 1 in]
        n23 = xnode "M_PWM"("Duty Cycle"="M_PWM", "Frequency [Hz]"=w111) -> ("error out"=w113:errorcluster)  [unwired: 1 in]
        n24 = Multiply(x="[cur] duty cycle [%] (s)", y=0.0001) -> (x*y=w139:dbl)
        n25 = Merge Errors(w113, w112, w185, w103) -> (w135:errorcluster)
        n26 = call <vilib>:"Set Duty Cycle and Frequency.vi"("error in (no error)"=w135, "Frequency [Hz]"=50.0 ("freq [Hz]"), "Duty Cycle"=w139, "PWM Ref In"=w136) -> ("error out"=w131:errorcluster, "PWM Ref Out"=w133:T19)  [unwired: 5 in]
        n27 = call <vilib>:"Read.vi"("error in (no error)"=w103, "Reset Counter"="Reset L_enc", "Encoder Ref In"=w105) -> ("error out"=w101:errorcluster, "Counter Value"=→"L_enc_value":i32, "Encoder Ref Out"=w99:T13)  [unwired: 4 in, 2 out]
        n28 = call <vilib>:"Read.vi"("error in (no error)"=w103, "Reset Counter"="Reset R_enc", "Encoder Ref In"=w104) -> ("error out"=w100:errorcluster, "Counter Value"=→"R_enc_value":i32, "Encoder Ref Out"=w98:T13)  [unwired: 4 in, 2 out]
        n29 = Merge Errors(w135, w101, w100) -> (w102:errorcluster)
        n30 = Multiply(x="[cur] duty cycle [%] (m)", y=0.0001) -> (x*y=w143:dbl)
        n31 = call <vilib>:"Set Duty Cycle and Frequency.vi"("error in (no error)"=w102, "Frequency [Hz]"=50.0 ("freq [Hz]"), "Duty Cycle"=w143, "PWM Ref In"=w120) -> ("error out"=w126:errorcluster, "PWM Ref Out"=w132:T19)  [unwired: 5 in]
        n32 = call <vilib>:"Read.vi"("error in (no error)"=w126, "Reset Counter"="Reset M_enc", "Encoder Ref In"=w122) -> ("error out"=w125:errorcluster, "Counter Value"=→"M_enc_value":i32, "Encoder Ref Out"=w119:T13)  [unwired: 4 in, 2 out]
        n33 = call <vilib>:"Read.vi"("Reset Counter"="Reset G_enc", "Encoder Ref In"=w121) -> ("Counter Value"=→"G_enc_value":i32, "Encoder Ref Out"=w118:T13)  [unwired: 5 in, 3 out]
        n34 = Wait Until Next ms Multiple(millisecond multiple=u32 25) -> ()  [unwired: 1 out]
        n35 = Merge Errors(w131, w126) -> (w134:errorcluster)
        n36 = call "dequeue_state.vi"("stop"="Stop", "error in (no error)"=w191, "queue in"=w174) -> ("error out"=w192:errorcluster, "state"=w187:T12, "queue out"=w176:refnum<queue>)  [unwired: 6 in]
        n37 = case shown="\"(auto) Analyze balls\"" w187 {
          tunnel: w192 -> [w463 w507 w514 w518 w525 w534 w538 w585 w660 w700 w718 w735 w745 w762 w792 w825 w831 w862 w880 w885 w901 w907 w956 w962 w998 w1016 w1084 w1111 w1117 w1133 w1141 w1151 w1177 w1265 w1306 w1313 w1318 w1322]
          tunnel: w176 -> [w464 _ _ _ w532 _ _ _ _ _ _ _ _ _ _ _ w830 _ _ _ _ _ _ _ _ _ _ _ _ _ _ _ _ _ _ _ _ _]
          tunnel: [w458 w491 w514 w518 w524 w534 w537 w585 w660 w700 w718 w735 w745 w762 w792 w825 w831 w862 w880 w885 w901 w907 w956 w961 w998 w1016 w1084 w1111 w1117 w1133 w1141 w1151 w1176 w1265 w1307 w1312 w1317 w1322] -> w164
          tunnel: w175 -> [w462 w502 w516 w520 w528 w533 w540 w582 w663 w693 w720 w728 w750 w775 w800 w827 w833 w856 w869 w898 w905 w913 w952 w964 w1000 w1017 w1094 w1113 w1128 w1131 w1140 w1155 w1175 w1257 w1309 w1315 w1320 w1326]
          tunnel: w94 -> [w465 w499 w517 w522 w531 w536 w542 w586 w664 w702 w723 w732 w751 w776 w803 w824 w835 w864 w865 w899 w906 w914 w955 w960 w1003 w1020 w1095 w1114 w1129 w1135 w1145 w1156 w1170 w1267 w1310 w1316 w1321 w1324]
          tunnel: [w465 w500 w517 w521 w531 w536 w542 w586 w664 w703 w723 w731 w751 w776 w802 w824 w834 w864 w879 w887 w906 w914 w954 w959 w1003 w1020 w1095 w1114 w1129 w1135 w1145 w1156 w1169 w1267 w1310 w1316 w1321 w1324] -> w95
          tunnel: "mode buttons" -> [_ _ _ _ _ _ _ _ _ _ w722 _ _ _ _ _ _ _ _ _ _ _ _ _ _ _ _ _ _ _ _ _ _ _ _ _ _ _]
          tunnel: [w462 w502 w516 w520 w528 w533 w540 w582 w663 w693 w720 w728 w750 w775 w800 w827 w832 w856 w871 w898 w905 w913 w952 w964 w1002 w1019 w1094 w1113 w1128 w1130 w1140 w1155 w1165 w1256 w1309 w1315 w1320 w1326] -> w97
          tunnel: [_ _ _ _ TRUE _ _ _ _ _ _ _ _ _ _ _ _ _ _ _ _ _ _ _ _ _ w1082 _ _ _ _ _ _ _ _ _ _ _] -> w173
          tunnel: w130 -> [w459 w497 w515 w519 w526 w535 w539 w581 w662 w697 w719 w727 w746 w763 w790 w826 w829 w863 w866 w886 w902 w908 w946 w963 w999 w1018 w1089 w1112 w1118 w1134 w1144 w1154 w1180 w1266 w1308 w1314 w1319 w1323]
          tunnel: [w459 w497 w515 w519 w526 w535 w539 w581 w662 w697 w719 w727 w746 w763 w790 w826 w829 w863 w866 w886 w902 w908 w946 w963 w999 w1018 w1093 w1112 w1118 w1134 w1144 w1154 w1180 w1258 w1308 w1314 w1319 w1323] -> w129
          tunnel: w119 -> [_ _ _ _ _ _ _ _ _ _ _ _ _ _ _ _ _ w861 _ _ _ _ _ _ _ _ _ _ _ _ w1143 _ _ w1262 _ _ _ _]
          tunnel: w118 -> [_ _ _ _ _ _ _ _ _ _ _ _ _ _ _ _ _ w860 _ _ _ _ _ _ _ _ _ _ _ _ w1142 _ _ w1261 _ _ _ _]
          tunnel: w99 -> [_ _ _ _ _ _ _ _ _ _ _ _ _ _ _ _ _ _ _ _ _ _ _ _ _ _ _ _ _ _ _ _ _ w1264 _ _ _ _]
          tunnel: w98 -> [_ _ _ _ _ _ _ _ _ _ _ _ _ _ _ _ _ _ _ _ _ _ _ _ _ _ _ _ _ _ _ _ _ w1263 _ _ _ _]
          frame "(qsm) schedule" {
            # "action buttons"
            # "Schedule tasks -- Use a selector tree (illustrated below), case structures, or other logic to specify state sequences (\"tasks\") to be performed in response to front-panel action buttons and flags set or cleared in other states."
            n38 = Unbundle By Name(w462) -> ("State"=w461:T1)
            n39 = case shown="\"Align\", Default" w461 {
              tunnel: [w467 w468 w469 w471 w472 _ _ _ _ _ _ _ _ _ w473 w474 w475 w476 w477 w478 w479 w480 w481 w482 w483 w485 w486 w487 w488 w490] -> w460
              frame "Align", Default {
                w467 = T33 [enum."Setup get", enum."Setup manipulator", enum."(image) get", enum."(image) show", enum."(ball) Align", enum."(ball) Wait", enum."(auto) Count balls", enum."(auto) Analyze balls", enum."(myRIO) update ports"] items=["(qsm) schedule", "(qsm) initialize", "(qsm) release", "(qsm) clean up", "(qsm) shutdown", "(myRIO) initialize", "(myRIO) clean up", "(myRIO) update ports", "Setup get", "(image) get", "(image) show", "(ball) Shape detection", "(ball) Calc ball indx", "(ball) Calculate ROI", "(ball) Analyze color", "(ball) Align", "(ball) Wait", "(ball) Grab", "(pattern) Find Square", "(pattern) Calculate ROI", "(pattern) Calc pattern indx", "Compare", "(pattern) Analyze pattern", "(pattern) Align", "(pattern) Wait", "(pattern) states control", "navx", "stop motors", "(joystick) Joystick control", "_Timer", "Setup manipulator", "(auto) Count balls", "(auto) Analyze balls", "(auto) Dot Controller", "(auto) Fwd (cm)", "(auto) Turn (angle)", "(auto) Tnl (M2-M2.5)", "Wait for button"]
                n40 = local write "Manip state"(enum16{"Align", "Grab", "Release"}."Align" ("Manip state")) -> ()
              }
              frame "1" {
                w468 = T33 [enum."Setup get", enum."(pattern) Align", enum."(auto) Fwd (cm)", enum."(myRIO) update ports", enum."(auto) Dot Controller"] items=["(qsm) schedule", "(qsm) initialize", "(qsm) release", "(qsm) clean up", "(qsm) shutdown", "(myRIO) initialize", "(myRIO) clean up", "(myRIO) update ports", "Setup get", "(image) get", "(image) show", "(ball) Shape detection", "(ball) Calc ball indx", "(ball) Calculate ROI", "(ball) Analyze color", "(ball) Align", "(ball) Wait", "(ball) Grab", "(pattern) Find Square", "(pattern) Calculate ROI", "(pattern) Calc pattern indx", "Compare", "(pattern) Analyze pattern", "(pattern) Align", "(pattern) Wait", "(pattern) states control", "navx", "stop motors", "(joystick) Joystick control", "_Timer", "Setup manipulator", "(auto) Count balls", "(auto) Analyze balls", "(auto) Dot Controller", "(auto) Fwd (cm)", "(auto) Turn (angle)", "(auto) Tnl (M2-M2.5)", "Wait for button"]
              }
              frame "2" {
                w469 = T33 [enum."Setup get", enum."(pattern) Align", enum."(auto) Turn (angle)", enum."(myRIO) update ports", enum."(auto) Dot Controller"] items=["(qsm) schedule", "(qsm) initialize", "(qsm) release", "(qsm) clean up", "(qsm) shutdown", "(myRIO) initialize", "(myRIO) clean up", "(myRIO) update ports", "Setup get", "(image) get", "(image) show", "(ball) Shape detection", "(ball) Calc ball indx", "(ball) Calculate ROI", "(ball) Analyze color", "(ball) Align", "(ball) Wait", "(ball) Grab", "(pattern) Find Square", "(pattern) Calculate ROI", "(pattern) Calc pattern indx", "Compare", "(pattern) Analyze pattern", "(pattern) Align", "(pattern) Wait", "(pattern) states control", "navx", "stop motors", "(joystick) Joystick control", "_Timer", "Setup manipulator", "(auto) Count balls", "(auto) Analyze balls", "(auto) Dot Controller", "(auto) Fwd (cm)", "(auto) Turn (angle)", "(auto) Tnl (M2-M2.5)", "Wait for button"]
              }
              frame "3" {
                w471 = T33 [enum."Setup get", enum."Setup manipulator", enum."(auto) Tnl (M2-M2.5)", enum."(myRIO) update ports", enum."(auto) Dot Controller"] items=["(qsm) schedule", "(qsm) initialize", "(qsm) release", "(qsm) clean up", "(qsm) shutdown", "(myRIO) initialize", "(myRIO) clean up", "(myRIO) update ports", "Setup get", "(image) get", "(image) show", "(ball) Shape detection", "(ball) Calc ball indx", "(ball) Calculate ROI", "(ball) Analyze color", "(ball) Align", "(ball) Wait", "(ball) Grab", "(pattern) Find Square", "(pattern) Calculate ROI", "(pattern) Calc pattern indx", "Compare", "(pattern) Analyze pattern", "(pattern) Align", "(pattern) Wait", "(pattern) states control", "navx", "stop motors", "(joystick) Joystick control", "_Timer", "Setup manipulator", "(auto) Count balls", "(auto) Analyze balls", "(auto) Dot Controller", "(auto) Fwd (cm)", "(auto) Turn (angle)", "(auto) Tnl (M2-M2.5)", "Wait for button"]
                n41 = local write "Manip state"(enum16{"Align", "Grab", "Release"}."Release" ("Manip state")) -> ()
              }
              frame "4" {
                w472 = T33 [enum."_Timer"] items=["(qsm) schedule", "(qsm) initialize", "(qsm) release", "(qsm) clean up", "(qsm) shutdown", "(myRIO) initialize", "(myRIO) clean up", "(myRIO) update ports", "Setup get", "(image) get", "(image) show", "(ball) Shape detection", "(ball) Calc ball indx", "(ball) Calculate ROI", "(ball) Analyze color", "(ball) Align", "(ball) Wait", "(ball) Grab", "(pattern) Find Square", "(pattern) Calculate ROI", "(pattern) Calc pattern indx", "Compare", "(pattern) Analyze pattern", "(pattern) Align", "(pattern) Wait", "(pattern) states control", "navx", "stop motors", "(joystick) Joystick control", "_Timer", "Setup manipulator", "(auto) Count balls", "(auto) Analyze balls", "(auto) Dot Controller", "(auto) Fwd (cm)", "(auto) Turn (angle)", "(auto) Tnl (M2-M2.5)", "Wait for button"]
              }
              frame "5" {
              }
              frame "6" {
              }
              frame "7" {
              }
              frame "8" {
              }
              frame "9" {
              }
              frame "10" {
              }
              frame "11" {
              }
              frame "12" {
              }
              frame "13" {
              }
              frame "(pattern) Align" {
                w473 = T33 [enum."Setup get", enum."(image) get", enum."(pattern) Find Square", enum."(pattern) Align", enum."(pattern) Wait", enum."(myRIO) update ports"] items=["(qsm) schedule", "(qsm) initialize", "(qsm) release", "(qsm) clean up", "(qsm) shutdown", "(myRIO) initialize", "(myRIO) clean up", "(myRIO) update ports", "Setup get", "(image) get", "(image) show", "(ball) Shape detection", "(ball) Calc ball indx", "(ball) Calculate ROI", "(ball) Analyze color", "(ball) Align", "(ball) Wait", "(ball) Grab", "(pattern) Find Square", "(pattern) Calculate ROI", "(pattern) Calc pattern indx", "Compare", "(pattern) Analyze pattern", "(pattern) Align", "(pattern) Wait", "(pattern) states control", "navx", "stop motors", "(joystick) Joystick control", "_Timer", "Setup manipulator", "(auto) Count balls", "(auto) Analyze balls", "(auto) Dot Controller", "(auto) Fwd (cm)", "(auto) Turn (angle)", "(auto) Tnl (M2-M2.5)", "Wait for button"] ("task")
              }
              frame "Pattern" {
                w474 = T33 [enum."Setup get", enum."(image) get", enum."(pattern) Find Square", enum."(pattern) Calculate ROI", enum."(pattern) Calc pattern indx", enum."(pattern) Analyze pattern", enum."(image) show", enum."(myRIO) update ports", enum."Wait for button"] items=["(qsm) schedule", "(qsm) initialize", "(qsm) release", "(qsm) clean up", "(qsm) shutdown", "(myRIO) initialize", "(myRIO) clean up", "(myRIO) update ports", "Setup get", "(image) get", "(image) show", "(ball) Shape detection", "(ball) Calc ball indx", "(ball) Calculate ROI", "(ball) Analyze color", "(ball) Align", "(ball) Wait", "(ball) Grab", "(pattern) Find Square", "(pattern) Calculate ROI", "(pattern) Calc pattern indx", "Compare", "(pattern) Analyze pattern", "(pattern) Align", "(pattern) Wait", "(pattern) states control", "navx", "stop motors", "(joystick) Joystick control", "_Timer", "Setup manipulator", "(auto) Count balls", "(auto) Analyze balls", "(auto) Dot Controller", "(auto) Fwd (cm)", "(auto) Turn (angle)", "(auto) Tnl (M2-M2.5)", "Wait for button"] ("task")
              }
              frame "(mod) pattern" {
                w475 = T33 [enum."Setup get", enum."_Timer", enum."(image) get", enum."(pattern) Find Square", enum."(pattern) Calculate ROI", enum."(pattern) Analyze pattern", enum."Compare", enum."(pattern) Calc pattern indx", enum."(image) show", enum."(myRIO) update ports", enum."Wait for button"] items=["(qsm) schedule", "(qsm) initialize", "(qsm) release", "(qsm) clean up", "(qsm) shutdown", "(myRIO) initialize", "(myRIO) clean up", "(myRIO) update ports", "Setup get", "(image) get", "(image) show", "(ball) Shape detection", "(ball) Calc ball indx", "(ball) Calculate ROI", "(ball) Analyze color", "(ball) Align", "(ball) Wait", "(ball) Grab", "(pattern) Find Square", "(pattern) Calculate ROI", "(pattern) Calc pattern indx", "Compare", "(pattern) Analyze pattern", "(pattern) Align", "(pattern) Wait", "(pattern) states control", "navx", "stop motors", "(joystick) Joystick control", "_Timer", "Setup manipulator", "(auto) Count balls", "(auto) Analyze balls", "(auto) Dot Controller", "(auto) Fwd (cm)", "(auto) Turn (angle)", "(auto) Tnl (M2-M2.5)", "Wait for button"] ("task")
              }
              frame "<mod>[P] remembering" {
                w476 = T33 [enum."Setup get", enum."_Timer", enum."(image) get", enum."(pattern) Find Square", enum."(pattern) Calculate ROI", enum."(pattern) Analyze pattern", enum."(pattern) Calc pattern indx", enum."(image) show", enum."(myRIO) update ports", enum."Wait for button", enum."(pattern) states control"] items=["(qsm) schedule", "(qsm) initialize", "(qsm) release", "(qsm) clean up", "(qsm) shutdown", "(myRIO) initialize", "(myRIO) clean up", "(myRIO) update ports", "Setup get", "(image) get", "(image) show", "(ball) Shape detection", "(ball) Calc ball indx", "(ball) Calculate ROI", "(ball) Analyze color", "(ball) Align", "(ball) Wait", "(ball) Grab", "(pattern) Find Square", "(pattern) Calculate ROI", "(pattern) Calc pattern indx", "Compare", "(pattern) Analyze pattern", "(pattern) Align", "(pattern) Wait", "(pattern) states control", "navx", "stop motors", "(joystick) Joystick control", "_Timer", "Setup manipulator", "(auto) Count balls", "(auto) Analyze balls", "(auto) Dot Controller", "(auto) Fwd (cm)", "(auto) Turn (angle)", "(auto) Tnl (M2-M2.5)", "Wait for button"] ("task")
              }
              frame "<mod>[P] go through tunnel" {
                w477 = T33 [enum."Setup get", enum."_Timer", enum."(image) get", enum."(pattern) Find Square", enum."(pattern) Calculate ROI", enum."(pattern) Analyze pattern", enum."(pattern) Calc pattern indx", enum."(image) show", enum."(myRIO) update ports", enum."Wait for button", enum."(pattern) states control"] items=["(qsm) schedule", "(qsm) initialize", "(qsm) release", "(qsm) clean up", "(qsm) shutdown", "(myRIO) initialize", "(myRIO) clean up", "(myRIO) update ports", "Setup get", "(image) get", "(image) show", "(ball) Shape detection", "(ball) Calc ball indx", "(ball) Calculate ROI", "(ball) Analyze color", "(ball) Align", "(ball) Wait", "(ball) Grab", "(pattern) Find Square", "(pattern) Calculate ROI", "(pattern) Calc pattern indx", "Compare", "(pattern) Analyze pattern", "(pattern) Align", "(pattern) Wait", "(pattern) states control", "navx", "stop motors", "(joystick) Joystick control", "_Timer", "Setup manipulator", "(auto) Count balls", "(auto) Analyze balls", "(auto) Dot Controller", "(auto) Fwd (cm)", "(auto) Turn (angle)", "(auto) Tnl (M2-M2.5)", "Wait for button"] ("task")
              }
              frame "<mod>[P] comparing" {
                w478 = T33 [enum."Setup get", enum."_Timer", enum."(image) get", enum."(pattern) Find Square", enum."(qsm) schedule", enum."(pattern) Calculate ROI", enum."(pattern) Analyze pattern", enum."(pattern) Calc pattern indx", enum."(image) show", enum."(myRIO) update ports", enum."Wait for button", enum."(pattern) states control"] items=["(qsm) schedule", "(qsm) initialize", "(qsm) release", "(qsm) clean up", "(qsm) shutdown", "(myRIO) initialize", "(myRIO) clean up", "(myRIO) update ports", "Setup get", "(image) get", "(image) show", "(ball) Shape detection", "(ball) Calc ball indx", "(ball) Calculate ROI", "(ball) Analyze color", "(ball) Align", "(ball) Wait", "(ball) Grab", "(pattern) Find Square", "(pattern) Calculate ROI", "(pattern) Calc pattern indx", "Compare", "(pattern) Analyze pattern", "(pattern) Align", "(pattern) Wait", "(pattern) states control", "navx", "stop motors", "(joystick) Joystick control", "_Timer", "Setup manipulator", "(auto) Count balls", "(auto) Analyze balls", "(auto) Dot Controller", "(auto) Fwd (cm)", "(auto) Turn (angle)", "(auto) Tnl (M2-M2.5)", "Wait for button"] ("task")
              }
              frame "(mod) ball" {
                w479 = T33 [enum."(image) get", enum."(image) get", enum."(ball) Shape detection", enum."(ball) Calculate ROI", enum."(ball) Analyze color", enum."Compare", enum."(ball) Calc ball indx", enum."(image) show", enum."(myRIO) update ports", enum."Wait for button"] items=["(qsm) schedule", "(qsm) initialize", "(qsm) release", "(qsm) clean up", "(qsm) shutdown", "(myRIO) initialize", "(myRIO) clean up", "(myRIO) update ports", "Setup get", "(image) get", "(image) show", "(ball) Shape detection", "(ball) Calc ball indx", "(ball) Calculate ROI", "(ball) Analyze color", "(ball) Align", "(ball) Wait", "(ball) Grab", "(pattern) Find Square", "(pattern) Calculate ROI", "(pattern) Calc pattern indx", "Compare", "(pattern) Analyze pattern", "(pattern) Align", "(pattern) Wait", "(pattern) states control", "navx", "stop motors", "(joystick) Joystick control", "_Timer", "Setup manipulator", "(auto) Count balls", "(auto) Analyze balls", "(auto) Dot Controller", "(auto) Fwd (cm)", "(auto) Turn (angle)", "(auto) Tnl (M2-M2.5)", "Wait for button"] ("task")
              }
              frame "Ball" {
                w480 = T33 [enum."(image) get", enum."(ball) Shape detection", enum."(ball) Calculate ROI", enum."(ball) Calc ball indx", enum."(ball) Analyze color", enum."(image) show", enum."Wait for button", enum."(myRIO) update ports"] items=["(qsm) schedule", "(qsm) initialize", "(qsm) release", "(qsm) clean up", "(qsm) shutdown", "(myRIO) initialize", "(myRIO) clean up", "(myRIO) update ports", "Setup get", "(image) get", "(image) show", "(ball) Shape detection", "(ball) Calc ball indx", "(ball) Calculate ROI", "(ball) Analyze color", "(ball) Align", "(ball) Wait", "(ball) Grab", "(pattern) Find Square", "(pattern) Calculate ROI", "(pattern) Calc pattern indx", "Compare", "(pattern) Analyze pattern", "(pattern) Align", "(pattern) Wait", "(pattern) states control", "navx", "stop motors", "(joystick) Joystick control", "_Timer", "Setup manipulator", "(auto) Count balls", "(auto) Analyze balls", "(auto) Dot Controller", "(auto) Fwd (cm)", "(auto) Turn (angle)", "(auto) Tnl (M2-M2.5)", "Wait for button"] ("task")
              }
              frame "Other" {
                w481 = T33 [enum."(image) get", enum."(pattern) Find Square", enum."(pattern) Calculate ROI", enum."(pattern) Analyze pattern", enum."(image) show", enum."Wait for button", enum."(myRIO) update ports", enum."(image) get", enum."(ball) Shape detection", enum."(ball) Calculate ROI", enum."(ball) Analyze color", enum."(image) show", enum."Wait for button", enum."(myRIO) update ports"] items=["(qsm) schedule", "(qsm) initialize", "(qsm) release", "(qsm) clean up", "(qsm) shutdown", "(myRIO) initialize", "(myRIO) clean up", "(myRIO) update ports", "Setup get", "(image) get", "(image) show", "(ball) Shape detection", "(ball) Calc ball indx", "(ball) Calculate ROI", "(ball) Analyze color", "(ball) Align", "(ball) Wait", "(ball) Grab", "(pattern) Find Square", "(pattern) Calculate ROI", "(pattern) Calc pattern indx", "Compare", "(pattern) Analyze pattern", "(pattern) Align", "(pattern) Wait", "(pattern) states control", "navx", "stop motors", "(joystick) Joystick control", "_Timer", "Setup manipulator", "(auto) Count balls", "(auto) Analyze balls", "(auto) Dot Controller", "(auto) Fwd (cm)", "(auto) Turn (angle)", "(auto) Tnl (M2-M2.5)", "Wait for button"] ("task")
              }
              frame "Clear" {
                w482 = T33 [enum."Setup get", enum."(ball) Grab", enum."(qsm) shutdown", enum."(myRIO) update ports"] items=["(qsm) schedule", "(qsm) initialize", "(qsm) release", "(qsm) clean up", "(qsm) shutdown", "(myRIO) initialize", "(myRIO) clean up", "(myRIO) update ports", "Setup get", "(image) get", "(image) show", "(ball) Shape detection", "(ball) Calc ball indx", "(ball) Calculate ROI", "(ball) Analyze color", "(ball) Align", "(ball) Wait", "(ball) Grab", "(pattern) Find Square", "(pattern) Calculate ROI", "(pattern) Calc pattern indx", "Compare", "(pattern) Analyze pattern", "(pattern) Align", "(pattern) Wait", "(pattern) states control", "navx", "stop motors", "(joystick) Joystick control", "_Timer", "Setup manipulator", "(auto) Count balls", "(auto) Analyze balls", "(auto) Dot Controller", "(auto) Fwd (cm)", "(auto) Turn (angle)", "(auto) Tnl (M2-M2.5)", "Wait for button"] ("task")
              }
              frame "navx" {
                w483 = T33 [enum."(auto) Dot Controller"] items=["(qsm) schedule", "(qsm) initialize", "(qsm) release", "(qsm) clean up", "(qsm) shutdown", "(myRIO) initialize", "(myRIO) clean up", "(myRIO) update ports", "Setup get", "(image) get", "(image) show", "(ball) Shape detection", "(ball) Calc ball indx", "(ball) Calculate ROI", "(ball) Analyze color", "(ball) Align", "(ball) Wait", "(ball) Grab", "(pattern) Find Square", "(pattern) Calculate ROI", "(pattern) Calc pattern indx", "Compare", "(pattern) Analyze pattern", "(pattern) Align", "(pattern) Wait", "(pattern) states control", "navx", "stop motors", "(joystick) Joystick control", "_Timer", "Setup manipulator", "(auto) Count balls", "(auto) Analyze balls", "(auto) Dot Controller", "(auto) Fwd (cm)", "(auto) Turn (angle)", "(auto) Tnl (M2-M2.5)", "Wait for button"]
              }
              frame "(auto) Balls Analyze" {
                w485 = T33 [enum."Setup get", enum."Setup manipulator", enum."(image) get", enum."(ball) Shape detection", enum."(auto) Count balls", enum."(auto) Analyze balls", enum."(myRIO) update ports"] items=["(qsm) schedule", "(qsm) initialize", "(qsm) release", "(qsm) clean up", "(qsm) shutdown", "(myRIO) initialize", "(myRIO) clean up", "(myRIO) update ports", "Setup get", "(image) get", "(image) show", "(ball) Shape detection", "(ball) Calc ball indx", "(ball) Calculate ROI", "(ball) Analyze color", "(ball) Align", "(ball) Wait", "(ball) Grab", "(pattern) Find Square", "(pattern) Calculate ROI", "(pattern) Calc pattern indx", "Compare", "(pattern) Analyze pattern", "(pattern) Align", "(pattern) Wait", "(pattern) states control", "navx", "stop motors", "(joystick) Joystick control", "_Timer", "Setup manipulator", "(auto) Count balls", "(auto) Analyze balls", "(auto) Dot Controller", "(auto) Fwd (cm)", "(auto) Turn (angle)", "(auto) Tnl (M2-M2.5)", "Wait for button"] ("task")
                n42 = local write "Manip state"(enum16{"Align", "Grab", "Release"}."Align" ("Manip state")) -> ()
              }
              frame "(auto) Ball Analyze" {
                w486 = T33 [enum."(ball) Calculate ROI", enum."(ball) Analyze color", enum."(auto) Analyze balls"] items=["(qsm) schedule", "(qsm) initialize", "(qsm) release", "(qsm) clean up", "(qsm) shutdown", "(myRIO) initialize", "(myRIO) clean up", "(myRIO) update ports", "Setup get", "(image) get", "(image) show", "(ball) Shape detection", "(ball) Calc ball indx", "(ball) Calculate ROI", "(ball) Analyze color", "(ball) Align", "(ball) Wait", "(ball) Grab", "(pattern) Find Square", "(pattern) Calculate ROI", "(pattern) Calc pattern indx", "Compare", "(pattern) Analyze pattern", "(pattern) Align", "(pattern) Wait", "(pattern) states control", "navx", "stop motors", "(joystick) Joystick control", "_Timer", "Setup manipulator", "(auto) Count balls", "(auto) Analyze balls", "(auto) Dot Controller", "(auto) Fwd (cm)", "(auto) Turn (angle)", "(auto) Tnl (M2-M2.5)", "Wait for button"] ("task")
              }
              frame "Joystick control" {
                w487 = T33 [enum."(joystick) Joystick control", enum."(myRIO) update ports"] items=["(qsm) schedule", "(qsm) initialize", "(qsm) release", "(qsm) clean up", "(qsm) shutdown", "(myRIO) initialize", "(myRIO) clean up", "(myRIO) update ports", "Setup get", "(image) get", "(image) show", "(ball) Shape detection", "(ball) Calc ball indx", "(ball) Calculate ROI", "(ball) Analyze color", "(ball) Align", "(ball) Wait", "(ball) Grab", "(pattern) Find Square", "(pattern) Calculate ROI", "(pattern) Calc pattern indx", "Compare", "(pattern) Analyze pattern", "(pattern) Align", "(pattern) Wait", "(pattern) states control", "navx", "stop motors", "(joystick) Joystick control", "_Timer", "Setup manipulator", "(auto) Count balls", "(auto) Analyze balls", "(auto) Dot Controller", "(auto) Fwd (cm)", "(auto) Turn (angle)", "(auto) Tnl (M2-M2.5)", "Wait for button"]
              }
              frame "(pattern) Align <loop>" {
                w488 = T33 [enum."Setup get", enum."(image) get", enum."(pattern) Find Square", enum."(pattern) Align", enum."(pattern) Wait", enum."(myRIO) update ports"] items=["(qsm) schedule", "(qsm) initialize", "(qsm) release", "(qsm) clean up", "(qsm) shutdown", "(myRIO) initialize", "(myRIO) clean up", "(myRIO) update ports", "Setup get", "(image) get", "(image) show", "(ball) Shape detection", "(ball) Calc ball indx", "(ball) Calculate ROI", "(ball) Analyze color", "(ball) Align", "(ball) Wait", "(ball) Grab", "(pattern) Find Square", "(pattern) Calculate ROI", "(pattern) Calc pattern indx", "Compare", "(pattern) Analyze pattern", "(pattern) Align", "(pattern) Wait", "(pattern) states control", "navx", "stop motors", "(joystick) Joystick control", "_Timer", "Setup manipulator", "(auto) Count balls", "(auto) Analyze balls", "(auto) Dot Controller", "(auto) Fwd (cm)", "(auto) Turn (angle)", "(auto) Tnl (M2-M2.5)", "Wait for button"] ("task")
              }
              frame "(ball) Align <loop>" {
                w490 = T33 [enum."Setup get", enum."Setup manipulator", enum."(image) get", enum."(ball) Shape detection", enum."(ball) Align", enum."(ball) Wait", enum."(auto) Count balls", enum."(auto) Analyze balls", enum."(myRIO) update ports"] items=["(qsm) schedule", "(qsm) initialize", "(qsm) release", "(qsm) clean up", "(qsm) shutdown", "(myRIO) initialize", "(myRIO) clean up", "(myRIO) update ports", "Setup get", "(image) get", "(image) show", "(ball) Shape detection", "(ball) Calc ball indx", "(ball) Calculate ROI", "(ball) Analyze color", "(ball) Align", "(ball) Wait", "(ball) Grab", "(pattern) Find Square", "(pattern) Calculate ROI", "(pattern) Calc pattern indx", "Compare", "(pattern) Analyze pattern", "(pattern) Align", "(pattern) Wait", "(pattern) states control", "navx", "stop motors", "(joystick) Joystick control", "_Timer", "Setup manipulator", "(auto) Count balls", "(auto) Analyze balls", "(auto) Dot Controller", "(auto) Fwd (cm)", "(auto) Turn (angle)", "(auto) Tnl (M2-M2.5)", "Wait for button"]
                n43 = local write "Manip state"(enum16{"Align", "Grab", "Release"}."Align" ("Manip state")) -> ()
              }
            }
            n44 = call "enqueue_states.vi"("task"=w460, "error in"=w463, "queue in"=w464) -> ("error out"=w458:errorcluster)  [unwired: 6 in, 1 out]
          }
          frame "(qsm) initialize" {
            w505 = T34 0 items=["Grayscale (U8)", "Grayscale (I16)", "Grayscale (SGL)", "Complex (CSG)", "RGB (U32)", "HSL (U32)", "RGB (U64)", "Grayscale (U16)"] ("Image Type")
            # "Initialize -- Allocate memory for additional image buffers, if necessary, and perform other one-time initialization steps."
            n45 = flat-sequence {
              frame #0 {
                n46 = Initialize Array(0 ("element"), "Dots in total") -> (→"Angles" →"Left_enc" →"Right_enc" →"M_enc" →"G_enc":i32[])
                n47 = local read "States in total"() -> (w510:i32)
                n48 = Initialize Array(0 ("element"), w510) -> (→"FT_Angles" →"FT_Left_enc" →"FT_Right_enc" →"FT_M_enc" →"FT_G_enc":i32[])
              }
            }
            n49 = Initialize Array(30, 16) -> (w492:i32[])
            n50 = call "IMAQ Create"("Border Size"=3, "Image Name"="img0", "Image Type"=w505, "error in (no error)"=w507) -> ("New Image"=w503:T8, "error out"=w491:errorcluster)  [unwired: 1 in]
            n51 = Initialize Array(20, 16) -> (w495:i32[])
            n52 = Bundle By Name(cluster=w499, "image ref"=w503) -> (w501:T11)
            n53 = Bundle By Name(cluster=w501, "Color classes"=w495, "Pattern classes"=w492) -> (w500:T11)
          }
          frame "(qsm) release" {
            # "Release all front-panel action buttons."
          }
          frame "(qsm) clean up" {
            # "Set the \"Stop webcam\" flag"
            # "Clean up -- Set the \"Stop webcam flag\" and perform other necessary clean-up actions."
            n54 = Bundle By Name(cluster=w522, "qsm.Stop webcam"=TRUE) -> (w521:T11)
          }
          frame "(qsm) shutdown" {
            # "deallocate image buffer memory"
            # "stop the loop"
            # "Shutdown -- Release the state queue, free all image buffer memory, and stop the while-loop structure."
            n55 = Release Queue(queue=w532, error in (no error)=w525) -> (error out=w529:errorcluster)  [unwired: 1 in, 2 out]
            n56 = call "Imaq Dispose"("All Images? (No)"=TRUE, "error in (no error)"=w529) -> ("error out"=w524:errorcluster)  [unwired: 4 in]
          }
          frame "(myRIO) initialize" {
            # "Initialize (myRIO) -- Open channels, configure devices, send setup strings to peripherals, etc."
          }
          frame "(myRIO) clean up" {
            w541 = FALSE ("LED3")
            # "clear the onboard LEDs"
            # "Clean up (myRIO) -- Return myRIO devices and external peripherals to inactive states."
            n57 = xnode "LED 3"("LED0"=w541, "LED1"=w541, "LED2"=w541, "LED3"=w541, "error in (no error)"=w538) -> ("error out"=w537:errorcluster)
          }
          frame "(myRIO) update ports" {
            # "show the button state\non the onboard LEDs"
            # "set the flag"
            # "press the onboard button\nto set the \"save image\" flag"
            # "Update ports (myRIO) -- Read and write onboard devices and external peripherals."
            n58 = xnode "Button"("error in (no error)"=w585) -> ("Value"=w583:bool, "error out"=w584:errorcluster)
            n59 = xnode "LED"("LED0"=w583, "LED1"=w583, "LED2"=w583, "LED3"=w583, "error in (no error)"=w584) -> ()  [unwired: 1 out]
          }
          frame "Setup get" {
            n60 = Unbundle By Name(w663) -> ("State"=w661:T1)
            n61 = flat-sequence {
              tunnel: w661 -> [w665]
              frame #0 {
                n62 = case shown="\"1\"" w665 {
                  frame "Align", Default {
                    n63 = local write "Camera state"(enum16{"Fwd", "Pattern", "Ball"}."Ball" ("Camera state")) -> ()
                    "rotate" <- FALSE ("rotate")
                  }
                  frame "1" {
                    n64 = local write "Camera state"(enum16{"Fwd", "Pattern", "Ball"}."Pattern" ("Camera state")) -> ()
                  }
                  frame "2" {
                  }
                  frame "3" {
                    n65 = local write "Camera state"(enum16{"Fwd", "Pattern", "Ball"}."Ball" ("Camera state")) -> ()
                  }
                  frame "4" {
                    n66 = local write "Camera state"(enum16{"Fwd", "Pattern", "Ball"}."Ball" ("Camera state")) -> ()
                  }
                  frame "5" {
                  }
                  frame "6" {
                  }
                  frame "7" {
                  }
                  frame "8" {
                  }
                  frame "9" {
                  }
                  frame "10" {
                  }
                  frame "11" {
                  }
                  frame "12" {
                  }
                  frame "13" {
                  }
                  frame "(pattern) Align" {
                    n67 = local write "rotate"(TRUE ("rotate")) -> ()
                    n68 = local write "Camera state"(enum16{"Fwd", "Pattern", "Ball"}."Pattern" ("Camera state")) -> ()
                  }
                  frame "Pattern" {
                    n69 = local write "Camera state"(enum16{"Fwd", "Pattern", "Ball"}."Pattern" ("Camera state")) -> ()
                  }
                  frame "(mod) pattern" {
                    n70 = local write "Camera state"(enum16{"Fwd", "Pattern", "Ball"}."Pattern" ("Camera state")) -> ()
                  }
                  frame "<mod>[P] remembering" {
                    n71 = local write "Camera state"(enum16{"Fwd", "Pattern", "Ball"}."Pattern" ("Camera state")) -> ()
                  }
                  frame "<mod>[P] go through tunnel" {
                    n72 = local write "Camera state"(enum16{"Fwd", "Pattern", "Ball"}."Pattern" ("Camera state")) -> ()
                  }
                  frame "<mod>[P] comparing" {
                    n73 = local write "Camera state"(enum16{"Fwd", "Pattern", "Ball"}."Pattern" ("Camera state")) -> ()
                  }
                  frame "(mod) ball" {
                    n74 = local write "Camera state"(enum16{"Fwd", "Pattern", "Ball"}."Ball" ("Camera state")) -> ()
                  }
                  frame "Ball" {
                    n75 = local write "Camera state"(enum16{"Fwd", "Pattern", "Ball"}."Ball" ("Camera state")) -> ()
                  }
                  frame "Other" {
                  }
                  frame "Clear" {
                    n76 = local write "Camera state"(enum16{"Fwd", "Pattern", "Ball"}."Ball" ("Camera state")) -> ()
                  }
                  frame "navx" {
                  }
                  frame "(auto) Balls Analyze" {
                    n77 = local write "Camera state"(enum16{"Fwd", "Pattern", "Ball"}."Ball" ("Camera state")) -> ()
                    n78 = local write "rotate"(FALSE ("rotate")) -> ()
                  }
                  frame "(auto) Ball Analyze" {
                  }
                  frame "(pattern) Align <loop>" {
                  }
                  frame "(ball) Align <loop>" {
                  }
                  frame "Joystick control" {
                  }
                }
              }
              frame #1 {
                n79 = call "Setup camera (SubVI).vi"("M duty cycle [P]"="M duty cycle [P]", "S duty cycle [B]   in"="S duty cycle [B]", "M duty cycle [B]  in"="M duty cycle [B]", "S duty cycle [F]"="S duty cycle [F]", "M duty cycle [F]"="M duty cycle [F]", "Camera state"="Camera state", "S duty cycle [P]"="S duty cycle [P]") -> ("M duty cycle [B]  out"=w684:dbl, "S duty cycle [B]   out"=w685:dbl)  [unwired: 3 in]
                n80 = local write "[cur] duty cycle [%] (s)"(w685) -> ()
                n81 = local write "[cur] duty cycle [%] (m)"(w684) -> ()
              }
            }
          }
          frame "(image) get" {
            # "NOTE:\n1. Use NI-MAX to configure your webcam with the\n     *same* resolution (\"mode\") and attributes as those used \n     to develop your Vision Assistant script, especially if the\n     script depends on absolute ROIs, calibration images, template\n     images, background levels, etc.\n \n     Click \"Save\" to create or update the camera configuration files\n     on the target.\n\n2. Open the Vision Acquisition Express VI above and then\n     select \"Reset to Defaults\" to read the camera configuration\n     files created/updated by NI-MAX in the previous step."
            # "webcam image buffer is\ncreated during the first\ncall of the Vision\nAcquisition Express VI"
            # "Get image -- Retrieve a single webcam image frame and optionally flip the image right side up."
            n82 = call "Vision Acquisition"("error in"=w700) -> ("Image Out"=w698:T8, "error out"=w699:errorcluster)  [unwired: 24 in, 1 out]
            n83 = local read "rotate"() -> (w701:bool)
            n84 = case shown="True" w701 {
              tunnel: w698 -> [w712 w717]
              tunnel: [w712 w716] -> w696
              tunnel: w699 -> [w711 w714]
              tunnel: [w711 w715] -> w695
              frame False {
                # "use webcam image as-is"
              }
              frame True {
                # "rotate img for pattern"
                n85 = call "IMAQ Rotate"("error in (no error)"=w714, "Angle (degrees)"="Angle for pattern (degrees)", "Image Src"=w717) -> ("error out"=w715:errorcluster, "Image Dst Out"=w716:T8)  [unwired: 7 in]
              }
            }
            n86 = Unbundle By Name(w693) -> ("State"=w692:T1)
            n87 = case shown="\"Align\", Default" w692 {
              tunnel: w696 -> [w705 w710]
              tunnel: w695 -> [w704 w707]
              tunnel: [w705 w709] -> w694
              tunnel: [w704 w708] -> _
              frame "Align", Default {
              }
              frame "(pattern) Align" {
                n88 = call "IMAQ Rotate"("error in (no error)"=w707, "Angle (degrees)"="Angle for Align (degrees)", "Image Src"=w710) -> ("error out"=w708:errorcluster, "Image Dst Out"=w709:T8)  [unwired: 7 in]
              }
            }
            n89 = Bundle By Name(cluster=w702, "qsm.Webcam image ref"=w694) -> (w703:T11)
          }
          frame "(image) show" {
            # "Show image -- Select from among the available image buffers to show on the main image display; use a selector tree or case structure."
            n90 = Unbundle By Name "Unbundle By Name"(w722) -> ("show analyzed"=w721:bool)
            n91 = Unbundle By Name "Unbundle By Name"(w723) -> ("qsm.Analyzed image ref"=w726:T8, "qsm.Webcam image ref"=w725:T8)
            n92 = Select(t=w726, s=w721, f=w725) -> (s? t:f=→"image display":T8)
          }
          frame "(ball) Shape detection" {
            # "Shape detection"
            # "Expansion State A"
            n93 = Unbundle By Name(w732) -> ("qsm.Webcam image ref"=w734:T8)
            n94 = call "Vision Assistant"("Image In"=w734, "error in"=w735) -> ("Image Out"=w733:T8, "Circles Calibrated (Shape Detection 1)"=w729:T4, "Number of Matches (Shape Detection 1)"=→"Number of Matches (Shape Detection 1)":i32)  [unwired: 22 in, 1 out]
            "Circles Calibrated (Shape Detection 1)" <- w729
            n95 = disable-structure shown="Disabled" {
              disable-tunnel: w729 -> [w744 _]
              frame Disabled {
                n96 = Index Array(array=w744, index=0) -> (element=w742:T35)
                n97 = Unbundle By Name(w742) -> ("Position"=w741:cluster{"X":sgl, "Y":sgl}, "Radius"=→"CircleRadius":dbl)
                n98 = Unbundle(w741) -> ("X"=w740:sgl, "Y"=w739:sgl)
                n99 = To Double Precision Float(number=w740) -> (double precision float=→"curX":dbl)
                n100 = To Double Precision Float(number=w739) -> (double precision float=→"curY":dbl)
              }
              frame Enabled {
              }
            }
            n101 = Bundle By Name(cluster=w732, "qsm.Analyzed image ref"=w733) -> (w731:T11)
          }
          frame "(ball) Calc ball indx" {
            n102 = Unbundle By Name(w750) -> ("State"=w747:T1)
            n103 = Equal?(x=w747, y=T30."(mod) ball" ("Shape - t, Color - f")) -> (x = y?=w749:bool)
            n104 = case shown="True" w749 {
              frame False {
                n105 = local read "Circles Calibrated (Shape Detection 1)"() -> (w756:T4)
                n106 = control-ref of="Ball number"() -> (w758:refnum<vi>)
                n107 = control-ref of="Number of Matches (Shape Detection 1)"() -> (w759:refnum<vi>)
                n108 = local read "curX"() -> (w755:dbl)
                n109 = local read "curY"() -> (w754:dbl)
                n110 = To Single Precision Float(number=w755) -> (single precision float=w753:sgl)
                n111 = To Single Precision Float(number=w754) -> (single precision float=w752:sgl)
                n112 = call "Ball Index (SubVI).vi"("cur pos Y"=w752, "cur pos X"=w753, "Circles Calibrated (Shape Detection 1)"=w756, "Ball index"="Ball number", "reference in"=w758, "Digital in"=w759) -> ()  [unwired: 4 in]
              }
              frame True {
                n113 = local read "Ball number"() -> (w761:i32)
                n114 = Increment(x=w761) -> (x+1=w760:i32)
                n115 = local write "Ball number"(w760) -> ()
              }
            }
          }
          frame "(ball) Calculate ROI" {
            n116 = local read "Number of Matches (Shape Detection 1)"() -> (w773:i32)
            n117 = Greater Than 0?(x=w773) -> (x > 0?=w770:bool)
            n118 = local read "curX"() -> (w772:dbl)
            n119 = local read "curY"() -> (w771:dbl)
            n120 = control-ref of="CircleRadius"() -> ()  [unwired: 1 out]
            n121 = local read "ROI Descriptor COLOR"() -> (w764:T5)
            n122 = call "Ball ROI (SubVI).vi"("ROI Descriptor COLOR Mask"=w764, "divider (circle)"="divider (circle)", "curY"=w771, "curX"=w772, "Boolean"=w770) -> ("x1"=→"1x1 (circle)":i32, "y0"=→"1y0 (circle)":i32, "x0"=→"1x0 (circle)":i32, "ROI Descriptor COLOR Mask out"=w765:T5, "y1"=→"1y1 (circle)":i32)  [unwired: 2 in]
            n123 = local write "ROI Descriptor COLOR"(w765) -> ()
          }
          frame "(ball) Analyze color" {
            # "Color analyze"
            # "analyzed image buffer is\ncreated during the first\ncall of the Vision\nAssistant Express VI *only*\nwhen \"Create Destination\nImage\" option is enabled"
            # "Analyze image -- Analyze the webcam image with a Vision Assistant script."
            n124 = Unbundle By Name "Unbundle By Name"(w803) -> ("Color classes"=w797:i32[], "qsm.Webcam image ref"=w795:T8)
            n125 = call "Vision Assistant2"("Image In"=w795, "error in"=w792, "ROI Descriptor (Image Mask 1)"="ROI Descriptor COLOR", "ROI Descriptor (Color Classification 1)"="ROI Descriptor COLOR") -> ("Image Out"=w793:T8, "Classes (Color Classification 1)"=w794:string[])  [unwired: 21 in, 1 out]
            n126 = local read "(auto) balls counter"() -> (w796:i32)
            n127 = Index Array(array=w794, index=0) -> (element=w801:string)
            n128 = Decimal String To Number(string=w801) -> (number=w789:i32)  [unwired: 2 in, 1 out]
            "Color" <- w789
            n129 = Replace Array Subset(array=w797, new element=w789, index=w796) -> (w798:i32[])
            n130 = Bundle By Name "Bundle By Name"(cluster=w803, "qsm.Analyzed image ref"=w793, "Color class"=w789, "Color classes"=w798) -> (w802:T11)
            n131 = local read "1"() -> (w788:i32)
            n132 = local read "2"() -> (w787:i32)
            n133 = local read "3"() -> (w786:i32)
            n134 = local read "4"() -> (w785:i32)
            n135 = local read "5"() -> (w784:i32)
            n136 = Equal?(x=w788, y=w789) -> (x = y?=w779:bool)
            n137 = Equal?(x=w787, y=w789) -> (x = y?=w780:bool)
            n138 = Equal?(x=w786, y=w789) -> (x = y?=w781:bool)
            n139 = Equal?(x=w785, y=w789) -> (x = y?=w782:bool)
            n140 = Equal?(x=w784, y=w789) -> (x = y?=w783:bool)
            n141 = Build Array(w779, w780, w781, w782, w783) -> (w778:bool[])
            n142 = Or Array Elements(Boolean array=w778) -> (logical OR=→"Found Right Ball":bool)
          }
          frame "(ball) Align" {
            # "Align"
            # "Expansion State B"
            n143 = local read "Y is in range"() -> (w810:bool)
            n144 = local read "X is in range"() -> (w811:bool)
            n145 = local read "L_PWM"() -> (w806:dbl)
            n146 = local read "R_PWM"() -> (w805:dbl)
            n147 = local read "curX"() -> (w821:dbl)
            n148 = local read "curY"() -> (w818:dbl)
            n149 = call "Ball Align(SubVI).vi"("Align X - t, Y - f"="Align X - t, Y - f", "x is in range"=w811, "y is in range"=w810, "L_PWM"=w806, "R_PWM"=w805, "curX"=w821, "defY"="defY", "curY"=w818, "defX"="defX", "RangeY"="RangeY", "RangeX"="RangeX") -> ("x_is_in_range"=→"X is in range":bool, "y_is_in_range"=→"Y is in range":bool, "Align_X-t,Y-f"=w809:bool, "Boolean 4"=w815:bool, "Boolean"=w812:bool, "Boolean 3"=w814:bool, "Boolean 2"=w813:bool, "L_PWM out"=w808:dbl, "R_PWM out"=w807:dbl)  [unwired: 7 in, 1 out]
            n150 = local write "Align X - t, Y - f"(w809) -> ()
            n151 = local write "R_PWM"(w807) -> ()
            n152 = local write "L_PWM"(w808) -> ()
            n153 = local write "Right+"(w814) -> ()
            n154 = local write "Right-"(w813) -> ()
            n155 = local write "Left-"(w815) -> ()
            n156 = local write "Left+"(w812) -> ()
          }
          frame "(ball) Wait" {
            # "Expansion State D"
            n157 = flat-sequence {
              frame #0 {
                n158 = Wait (ms)(milliseconds to wait="align accuracy") -> ()  [unwired: 1 out]
              }
              frame #1 {
                w840 = FALSE
                n159 = local write "Left-"(w840) -> ()
                n160 = local write "Left+"(w840) -> ()
                n161 = local write "Right+"(w840) -> ()
                n162 = local write "Right-"(w840) -> ()
              }
            }
            n163 = local read "X is in range"() -> (w837:bool)
            n164 = local read "Y is in range"() -> (w836:bool)
            n165 = And(x=w837, y=w836) -> (x .and. y?=w838:bool)
            n166 = case shown="True" w838 {
              selector: w838 -> [w842 w853]
              tunnel: w835 -> [w848 w855]
              tunnel: [w848 w855] -> w834
              tunnel: w833 -> [w847 w850]
              tunnel: [w845 w849] -> w832
              tunnel: w831 -> [w846 w854]
              tunnel: [w846 w854] -> _
              tunnel: w830 -> [_ _]
              tunnel: [w842 w853] -> w828
              frame False {
                n167 = Unbundle(T9 {"State"=enum."Align"} ("Shape - t, Color - f")) -> ("State"=w843:T1)
                n168 = local write "Found Right Ball"(FALSE ("Found Right Ball")) -> ()
                n169 = Bundle By Name(cluster=w847, "State"=w843) -> (w845:T9)
              }
              frame True {
                n170 = Unbundle(T9 {"State"=enum."Clear"} ("Shape - t, Color - f")) -> ("State"=w851:T1)
                n171 = Bundle By Name(cluster=w850, "State"=w851) -> (w849:T9)
              }
            }
            "Ready to Grab" <- w828
          }
          frame "(ball) Grab" {
            # "Expansion State E"
            n172 = call "Setup manipulator (SubVI).vi"("Reverse?"=FALSE ("Release?"), "G_upper bound"="G_UB_grab", "M_lower bound"="M_UB_grab", "error in (no error)"=w862, "M_Encoder Ref In"=w861, "G_Encoder Ref In"=w860) -> ()  [unwired: 9 in, 1 out]
          }
          frame "(pattern) Find Square" {
            # "analyzed image buffer is\ncreated during the first\ncall of the Vision\nAssistant Express VI *only*\nwhen \"Create Destination\nImage\" option is enabled"
            # "Expansion State F"
            n173 = Unbundle By Name "Unbundle By Name"(w865) -> ("qsm.Webcam image ref"=w882:T8)
            n174 = call "Vision Assistant3"("Image In"=w882, "error in"=w880) -> ("Image Out"=w878:T8, "Calibrated Matches (Geometric Matching 1)"=w877:T6[], "Number of Matches (Geometric Matching 1)"=→"Number of Matches (Geometric Matching 1)":i32)  [unwired: 22 in, 1 out]
            "Calibrated Matches (Geometric Matching 1)" <- w877
            n175 = Bundle By Name(cluster=w865, "qsm.Analyzed image ref"=w878) -> (w879:T11)
            n176 = Index Array(array=w877, index=0) -> (element=w875:T6)
            n177 = Unbundle By Name(w875) -> ("Position"=w874:cluster{"x":sgl, "y":sgl})
            n178 = Unbundle By Name(w874) -> ("x"=→"curX(p)":sgl)
            n179 = Unbundle By Name(w869) -> ("State"=w868:T1)
            n180 = Equal?(x=w868, y=T31."<mod>[P] comparing") -> (x = y?=w872:bool)
            n181 = case shown="True" w872 {
              tunnel: [w883 T31."(pattern) Align" ("Shape - t, Color - f")] -> w870
              tunnel: w868 -> [w883 _]
              frame False {
              }
              frame True {
              }
            }
            n182 = Bundle By Name(cluster=w869, "State"=w870) -> (w871:T9)
          }
          frame "(pattern) Calculate ROI" {
            # "Expansion State G"
            n183 = local read "Number of Matches (Geometric Matching 1)"() -> (w897:i32)
            n184 = local read "Calibrated Matches (Geometric Matching 1)"() -> (w896:T6[])
            n185 = Unbundle By Name(w899) -> ("ROI Descriptor (Image Mask 1).Contours"=w889:T36)
            n186 = Greater Than 0?(x=w897) -> (x > 0?=w900:bool)
            n187 = call "Pattern ROI (SubVI).vi"("y"="divider (pattern)", "Boolean"=w900, "Calibrated Matches (Geometric Matching 1)"=w896, "Contours in"=w889) -> ("Numeric 4"=→"y1":i32, "Numeric 3"=→"x1":i32, "Numeric"=→"y0":i32, "Scale"=→"Scale":sgl, "Numeric 2"=→"x0":i32, "Contours out"=w888:T36)  [unwired: 2 in]
            n188 = Bundle By Name(cluster=w899, "ROI Descriptor (Image Mask 1).Contours"=w888) -> (w887:T11)
          }
          frame "(pattern) Calc pattern indx" {
            n189 = local read "pattern number"() -> (w904:i32)
            n190 = Increment(x=w904) -> (x+1=w903:i32)
            n191 = local write "pattern number"(w903) -> ()
          }
          frame "Compare" {
            n192 = Unbundle By Name(w913) -> ("State"=w912:T1)
            n193 = Equal?(x=w912, y=T32."(mod) ball") -> (x = y?=w910:bool)
            n194 = Not(x=w910) -> (.not. x?=w909:bool)
            n195 = case shown="False" w909 {
              tunnel: w914 -> [w918 w924]
              frame False {
                n196 = local read "Ball number"() -> (w919:i32)
                n197 = control-ref of="ball match"() -> (w916:refnum<vi>)
                n198 = Unbundle By Name(w918) -> ("Color classes"=w917:i32[])
                n199 = Greater?(x=w919, y="Balls to remember") -> (0:w921:bool)
                n200 = call "(ball) Compare (SubVI).vi"("Boolean"=w921, "Balls to remember"="Balls to remember", "Ball number"=w919, "Color classes"=w917, "Boolean in"=w916) -> ("ball match"=→"ball match":bool)  [unwired: 6 in]
              }
              frame True {
                n201 = local read "pattern number"() -> (w922:i32)
                n202 = Greater?(x=w922, y="patterns to remember") -> (0:w926:bool)
                n203 = Unbundle By Name(w924) -> ("Pattern classes"=w923:i32[])
                n204 = case shown="True" w926 {
                  tunnel: "patterns to remember" -> [_ w930]
                  tunnel: w923 -> [_ w928]
                  tunnel: w922 -> [_ w927]
                  frame False {
                  }
                  frame True {
                    n205 = flat-sequence {
                      tunnel: w930 -> [w932]
                      tunnel: [w932] -> w929
                      tunnel: w929 -> [w935]
                      tunnel: w928 -> [w934]
                      tunnel: w927 -> [w933]
                      frame #0 {
                        n206 = local write "pattern match"(FALSE ("pattern match")) -> ()
                      }
                      frame #1 {
                        n207 = for {
                          N: w935 -> [_]
                          tunnel: w933 -> [w944]
                          tunnel: w934 -> [w938]
                          i -> [w940]
                          n208 = Increment(x=w940) -> (x+1=w939:i32)
                          n209 = Index Array(array=w938, index=w939) -> (element=w937:i32)
                          n210 = Index Array(array=w938, index=w944) -> (element=w936:i32)
                          n211 = Equal?(x=w937, y=w936) -> (x = y?=w943:bool)
                          n212 = local read "pattern match"() -> (w942:bool)
                          n213 = Not(x=w942) -> (.not. x?=w941:bool)
                          n214 = case shown="True" w941 {
                            tunnel: w943 -> [_ w945]
                            frame False {
                            }
                            frame True {
                              "pattern match" <- w945
                            }
                          }
                        }
                      }
                    }
                  }
                }
              }
            }
          }
          frame "(pattern) Analyze pattern" {
            n215 = Unbundle By Name(w955) -> ("Pattern classes"=w949:i32[], "qsm.Webcam image ref"=w958:T8, "ROI Descriptor (Image Mask 1)"=w953:T5)
            n216 = call "Vision Assistant4"("Image In"=w958, "error in"=w956, "ROI Descriptor (Image Mask 1)"=w953, "ROI Descriptor (Particle Classification 1)"=w953) -> ("Image Out"=w957:T8, "Class (Particle Classification 1)"=w948:string)  [unwired: 21 in, 1 out]
            n217 = Decimal String To Number(string=w948) -> (number=w947:i32)  [unwired: 2 in, 1 out]
            "Pattern" <- w947
            n218 = Insert Into Array(array=w949, index="pattern number", new element=w947) -> (w951:i32[])
            n219 = Bundle By Name(cluster=w955, "qsm.Analyzed image ref"=w957, "Pattern classes"=w951) -> (w954:T11)
          }
          frame "(pattern) Align" {
            n220 = while {
              tunnel: w962 -> [w973]
              tunnel: [w971] -> w961
              shift-right: [w965] -> w959
              shift-left: w960 -> [w970]
              stop <- w976 stop-if-true
              n221 = flat-sequence {
                tunnel: [w980] -> w968
                tunnel: [w978] -> w974
                tunnel: w973 -> [w977]
                tunnel: [w987] -> w967
                tunnel: [w984] -> w975
                tunnel: w974 -> [w986]
                tunnel: [w985] -> w972
                tunnel: w969 -> [w983]
                tunnel: [w995] -> w976
                tunnel: w975 -> [w997]
                tunnel: w972 -> [w996]
                tunnel: [w996] -> w971
                frame #0 {
                  n222 = local read "Angle for pattern (degrees)"() -> (w981:sgl)
                  n223 = call "Vision Acquisition2"("error in"=w977) -> ("Image Out"=w982:T8, "error out"=w979:errorcluster)  [unwired: 24 in, 1 out]
                  n224 = call "IMAQ Rotate"("error in (no error)"=w979, "Angle (degrees)"=w981, "Image Dst"=w982, "Image Src"=w982) -> ("error out"=w978:errorcluster, "Image Dst Out"=w980:T8)  [unwired: 6 in]
                }
                frame #1 {
                  n225 = call "Vision Assistant6"("Image In"=w983, "error in"=w986) -> ("Image Out"=w987:T8, "error out"=w985:errorcluster, "Calibrated Matches (Geometric Matching 1)"=w988:T6[], "Number of Matches (Geometric Matching 1)"=w989:i32)  [unwired: 22 in]
                  n226 = Index Array(array=w988, index=0) -> (element=w991:T6)
                  n227 = local write "Number of Matches (Geometric Matching 1)"(w989) -> ()
                  n228 = local write "Calibrated Matches (Geometric Matching 1)"(w988) -> ()
                  n229 = Unbundle By Name(w991) -> ("Position"=w990:cluster{"x":sgl, "y":sgl})
                  n230 = Unbundle By Name(w990) -> ("x"=w984:sgl)
                  n231 = local write "curX(p)"(w984) -> ()
                }
                frame #2 {
                  n232 = call "Pattern Align(SubVI).vi"("curX(p)"=w997, "defX(p)"="defX(p)", "Range(p)"="Range(p)") -> ("In Range?"=w995:bool)  [unwired: 8 in]
                  "In Range? (p)" <- w995
                }
              }
              n233 = Bundle By Name(cluster=w970, "qsm.Webcam image ref"=w968) -> (w966:T11)
              n234 = Unbundle By Name(w966) -> ("qsm.Webcam image ref"=w969:T8)
              n235 = Bundle By Name(cluster=w966, "qsm.Analyzed image ref"=w967) -> (w965:T11)
            }
          }
          frame "(pattern) Wait" {
            n236 = flat-sequence {
              tunnel: [w1007] -> w1001
              tunnel: w1000 -> [w1006]
              frame #0 {
                n237 = Wait (ms)(milliseconds to wait="align accuracy (p)") -> ()  [unwired: 1 out]
              }
              frame #1 {
                w1005 = FALSE ("Right+")
                n238 = local write "Right+"(w1005) -> ()
                n239 = local write "Right-"(w1005) -> ()
                n240 = local write "Left+"(w1005) -> ()
                n241 = local write "Left-"(w1005) -> ()
              }
              frame #2 {
                n242 = local read "In Range? (p)"() -> (w1008:bool)
                n243 = Equal?(x=".Task", y=enum16{"Def", "<mod>[P]+tnl "}."<mod>[P]+tnl ") -> (x = y?=w1010:bool)
                n244 = And(x=w1008, y=w1010) -> (x .and. y?=w1009:bool)
                n245 = case shown="False" w1009 {
                  tunnel: [T31."(pattern) Align" ("Shape - t, Color - f") w1015] -> w1007
                  tunnel: w1006 -> [_ w1014]
                  frame False {
                  }
                  frame True {
                    n246 = Unbundle By Name(w1014) -> ("State"=w1015:T1)
                  }
                }
              }
            }
            n247 = Bundle By Name(cluster=w1000, "State"=w1001) -> (w1002:T9)
          }
          frame "(pattern) states control" {
            n248 = flat-sequence {
              tunnel: w1017 -> [w1025]
              tunnel: w1017 -> [w1024]
              tunnel: [w1023] -> w1019
              frame #0 {
                n249 = Increment(x=",ctl num") -> (x+1=w1021:i32)
                n250 = local write ",ctl num"(w1021) -> ()
              }
              frame #1 {
                n251 = Unbundle By Name(w1025) -> ("State"=w1026:T1)
                n252 = case shown="\"(ball) Align <loop>\"" w1026 {
                  tunnel: w1024 -> [w1029 w1039 w1049 w1055 w1056 w1057 w1058 w1059 w1060 w1061 w1062 w1063 w1064 w1065 w1066 w1067 w1068 w1069 w1070 w1071 w1072 w1073 w1074 w1075 w1076 w1077 w1078 w1079 w1080 w1081]
                  tunnel: [w1028 w1038 w1049 w1055 w1056 w1057 w1058 w1059 w1060 w1061 w1062 w1063 w1064 w1065 w1066 w1067 w1068 w1069 w1070 w1071 w1072 w1073 w1074 w1075 w1076 w1077 w1078 w1079 w1080 w1081] -> w1023
                  frame "<mod>[P] remembering" {
                    n253 = local read ",ctl num"() -> (w1031:i32)
                    n254 = Greater?(x=w1031, y=3) -> (0:w1027:bool)
                    n255 = case shown="True" w1027 {
                      tunnel: w1029 -> [w1032 w1037]
                      tunnel: [w1032 w1036] -> w1028
                      frame False {
                      }
                      frame True {
                        n256 = Unbundle(T9 {"State"=enum."<mod>[P] go through tunnel"} ("Shape - t, Color - f")) -> ("State"=w1033:T1)
                        n257 = Bundle By Name(cluster=w1037, "State"=w1033) -> (w1036:T9)
                        n258 = local write ",ctl num"(0 ("ctl num")) -> ()
                      }
                    }
                  }
                  frame "<mod>[P] go through tunnel" {
                    n259 = local read ",ctl num"() -> (w1042:i32)
                    n260 = Greater?(x=w1042, y=1) -> (0:w1040:bool)
                    n261 = case shown="True" w1040 {
                      tunnel: w1039 -> [w1043 w1048]
                      tunnel: [w1043 w1047] -> w1038
                      frame False {
                      }
                      frame True {
                        n262 = Unbundle(T9 {"State"=enum."<mod>[P] comparing"}) -> ("State"=w1044:T1)
                        n263 = Bundle By Name(cluster=w1048, "State"=w1044) -> (w1047:T9)
                        n264 = local write ",ctl num"(0 (",ctl num")) -> ()
                      }
                    }
                  }
                  frame "<mod>[P] comparing" {
                    n265 = local read ",ctl num"() -> (w1051:i32)
                    n266 = Greater?(x=w1051, y=5) -> (0:w1052:bool)
                    n267 = case shown="True" w1052 {
                      frame False {
                      }
                      frame True {
                        n268 = local write ",ctl num"(0 (",ctl num")) -> ()
                        n269 = local write "Stop"(TRUE ("Stop")) -> ()
                      }
                    }
                  }
                  frame "(mod) ball" {
                  }
                  frame "Ball" {
                  }
                  frame "Other" {
                  }
                  frame "Clear" {
                  }
                  frame "(auto) Balls Analyze" {
                  }
                  frame "(auto) Ball Analyze" {
                  }
                  frame "Joystick control" {
                  }
                  frame "(mod) pattern" {
                  }
                  frame "Pattern" {
                  }
                  frame "(pattern) Align" {
                  }
                  frame "Align" {
                  }
                  frame "navx" {
                  }
                  frame "1" {
                  }
                  frame "2" {
                  }
                  frame "3" {
                  }
                  frame "4" {
                  }
                  frame "5" {
                  }
                  frame "6" {
                  }
                  frame "7" {
                  }
                  frame "8" {
                  }
                  frame "9" {
                  }
                  frame "10" {
                  }
                  frame "11" {
                  }
                  frame "12" {
                  }
                  frame "13" {
                  }
                  frame "(pattern) Align <loop>" {
                  }
                  frame "(ball) Align <loop>" {
                  }
                }
              }
            }
          }
          frame "navx" {
            n270 = disable-structure shown="Disabled" {
              disable-tunnel: w1084 -> [w1100 _]
              disable-tunnel: [w1099 _] -> w1083
              disable-tunnel: [w1096 _] -> w1082
              frame Disabled {
                n271 = call "sonic info (SubVI).vi"("error in (no error)"=w1100) -> ("error out"=w1099:errorcluster, "distance to the side"=w1098:u32)  [unwired: 9 in]
                "distance to the side" <- w1098
                n272 = Less Or Equal?(x=w1098, y=u32 7) -> (x <= y?=w1096:bool)
              }
              frame Enabled {
              }
            }
            n273 = disable-structure shown="Disabled" {
              disable-tunnel: _ -> [w1110 _]
              disable-tunnel: _ -> [w1109 _]
              disable-tunnel: [w1108 _] -> _
              disable-tunnel: [w1102 _] -> _
              disable-tunnel: [w1101 _] -> _
              frame Disabled {
                n274 = control-ref of="Left+"() -> (w1107:refnum<vi>)
                n275 = control-ref of="Left-"() -> (w1106:refnum<vi>)
                n276 = control-ref of="Right+"() -> (w1105:refnum<vi>)
                n277 = control-ref of="Right-"() -> (w1104:refnum<vi>)
                n278 = call "align.vi"("Right-"=w1104, "I2C Ref Out"=w1110, "error in (no error)"=w1109, "Right+"=w1105, "Left-"=w1106, "Left+"=w1107) -> ("error out"=w1102:errorcluster, "Aligned"=w1101:bool, "value Z"=→"value Z":ext, "I2C Ref Out out"=w1108:T23)  [unwired: 2 in]
              }
              frame Enabled {
              }
            }
            n279 = control-ref of="L_PWM"() -> (w1092:refnum<vi>)
            n280 = control-ref of="R_PWM"() -> (w1091:refnum<vi>)
            n281 = call "fwd-navx (SubVI).vi"("error in (no error)"=w1083, "I2C Ref Out"=w1089, "R_PWM"=w1091, "L_PWM"=w1092) -> ("I2C Ref Out out"=w1093:T23, "value Z"=→"value Z 2":ext, "Right+"=w1088:bool, "Left+"=w1087:bool)  [unwired: 3 in, 1 out]
            n282 = Not(x=w1087) -> (.not. x?=w1086:bool)
            n283 = Not(x=w1088) -> (.not. x?=w1085:bool)
            n284 = local write "Left+"(w1087) -> ()
            n285 = local write "Left-"(w1086) -> ()
            n286 = local write "Right+"(w1088) -> ()
            n287 = local write "Right-"(w1085) -> ()
          }
          frame "stop motors" {
            n288 = flat-sequence {
              frame #0 {
                w1115 = TRUE ("Right+")
                n289 = local write "Left+"(w1115) -> ()
                n290 = local write "Left-"(w1115) -> ()
                n291 = local write "Right+"(w1115) -> ()
                n292 = local write "Right-"(w1115) -> ()
              }
              frame #1 {
                w1116 = FALSE ("Right+")
                n293 = local write "Left+"(w1116) -> ()
                n294 = local write "Left-"(w1116) -> ()
                n295 = local write "Right+"(w1116) -> ()
                n296 = local write "Right-"(w1116) -> ()
              }
            }
          }
          frame "(joystick) Joystick control" {
            n297 = shared-variable "My Computer\\KeyLibrary.lvlib\\Power"() -> (w1119:dbl)  [unwired: 1 in, 1 out]
            n298 = call "Joystick control (SubVI).vi"() -> ("G+"=w1125:bool, "M-"=w1127:bool, "M+"=w1126:bool, "G-"=w1124:bool, "Left+"=w1121:bool, "Right-"=w1120:bool, "Left-"=w1122:bool, "Right+"=w1123:bool)  [unwired: 4 in]
            n299 = local write "L_PWM"(w1119) -> ()
            n300 = local write "R_PWM"(w1119) -> ()
            n301 = local write "M-"(w1124) -> ()
            n302 = local write "G+"(w1126) -> ()
            n303 = local write "Right+"(w1123) -> ()
            n304 = local write "Right-"(w1120) -> ()
            n305 = local write "Left+"(w1121) -> ()
            n306 = local write "Left-"(w1122) -> ()
            n307 = local write "G-"(w1127) -> ()
            n308 = local write "M+"(w1125) -> ()
          }
          frame "_Timer" {
            n309 = Bundle By Name(cluster=w1131, "State"=T1."Align") -> (w1130:T9)
          }
          frame "Setup manipulator" {
            n310 = case shown="\"Release\"" "Manip state" {
              tunnel: ["G_UB_Align" w1148 w1150] -> w1138
              tunnel: ["M_UB_Align" w1149 w1150] -> w1139
              frame "Align", Default {
              }
              frame "Grab" {
                n311 = local read "M_UB_grab"() -> (w1149:i32)
                n312 = local read "G_UB_grab"() -> (w1148:i32)
              }
              frame "Release" {
                w1150 = 0
              }
            }
            n313 = call "Setup manipulator (SubVI).vi"("Reverse?"=FALSE ("Release?"), "G_upper bound"=w1138, "M_lower bound"=w1139, "error in (no error)"=w1141, "M_Encoder Ref In"=w1143, "G_Encoder Ref In"=w1142) -> ()  [unwired: 9 in, 1 out]
          }
          frame "(auto) Count balls" {
            n314 = local read "Circles Calibrated (Shape Detection 1)"() -> (w1152:T4)
            n315 = call "(auto) Count balls (SubVI).vi"("error in"=w1151, "Circles Calibrated (Shape Detection 1)"=w1152) -> ("balls counter"=→"(auto) balls counter":i32)  [unwired: 8 in, 1 out]
          }
          frame "(auto) Analyze balls" {
            n316 = call "Vision Acquisition3"() -> ()  [unwired: 25 in, 3 out]
            n317 = local read "(auto) balls counter"() -> (w1179:i32)
            n318 = local write "Number of Matches (Shape Detection 1)"(w1160) -> ()
            n319 = flat-sequence {
              tunnel: w1179 -> [w1195]
              tunnel: w1159 -> [w1194]
              tunnel: [w1193] -> w1178
              tunnel: w1177 -> [w1192]
              tunnel: [w1191] -> w1176
              tunnel: [w1190] -> w1171
              tunnel: [w1189] -> w1168
              tunnel: [w1188] -> w1167
              tunnel: w1158 -> [w1187]
              tunnel: w1161 -> [w1186]
              tunnel: [w1185] -> w1160
              tunnel: [w1246] -> w1163
              tunnel: w1175 -> [w1245]
              tunnel: w1168 -> [w1242]
              tunnel: w1167 -> [w1241]
              frame #0 {
                n320 = for {
                  N: w1195 -> [_]
                  tunnel: w1194 -> [w1207]
                  tunnel: [w1206] -> w1193
                  tunnel: w1192 -> [w1205]
                  tunnel: [w1204] -> w1191
                  tunnel: [w1200] -> w1190
                  tunnel: [w1199] -> w1189
                  tunnel: [w1198] -> w1188
                  tunnel: w1187 -> [w1196]
                  tunnel: w1186 -> [w1197]
                  tunnel: [w1197] -> w1185
                  i -> [w1202]
                  stop <- w1201 stop-if-true
                  n321 = flat-sequence {
                    tunnel: w1207 -> [w1227]
                    tunnel: [w1226] -> w1206
                    tunnel: w1205 -> [w1223]
                    tunnel: [w1222] -> w1204
                    tunnel: [w1214] -> w1203
                    tunnel: w1202 -> [_]
                    tunnel: [w1214] -> w1200
                    tunnel: [w1212] -> w1199
                    tunnel: [w1213] -> w1198
                    tunnel: w1196 -> [w1209]
                    tunnel: w1197 -> [w1208]
                    tunnel: w1203 -> [w1229]
                    tunnel: [w1228] -> w1201
                    frame #0 {
                      n322 = Index Array(array=w1209) -> (element=w1216:T35)  [unwired: 1 in]
                      n323 = Unbundle(w1216) -> ("Position"=w1215:cluster{"X":sgl, "Y":sgl}, "Radius"=w1211:dbl)  [unwired: 1 out]
                      n324 = local read "ROI Descriptor COLOR"() -> (w1225:T5)
                      n325 = Unbundle(w1215) -> ("X"=w1212:sgl, "Y"=w1213:sgl)
                      n326 = local read "divider (circle)"() -> (w1210:dbl)
                      n327 = Greater Than 0?(x=w1208) -> (x > 0?=w1217:bool)
                      n328 = call "Analyze ball (SubVI).vi"("ROI Descriptor COLOR Mask"=w1225, "Radius"=w1211, "Boolean"=w1217, "curX"=w1212, "curY"=w1213, "divider (circle)"=w1210, "Image In"=w1227, "error in"=w1223) -> ("Color"=w1214:i32, "Image Out"=w1226:T8, "error out"=w1222:errorcluster, "ROI Descriptor COLOR Mask out"=w1224:T5, "x0"=w1221:i32, "y0"=w1220:i32, "x1"=w1219:i32, "y1"=w1218:i32)  [unwired: 4 in]
                      n329 = local write "ROI Descriptor COLOR"(w1224) -> ()
                      n330 = local write "Color"(w1214) -> ()
                      n331 = local write "1x0 (circle)"(w1221) -> ()
                      n332 = local write "1x1 (circle)"(w1219) -> ()
                      n333 = local write "1y0 (circle)"(w1220) -> ()
                      n334 = local write "1y1 (circle)"(w1218) -> ()
                    }
                    frame #1 {
                      n335 = local read "1"() -> (w1234:i32)
                      n336 = local read "2"() -> (w1233:i32)
                      n337 = local read "3"() -> (w1232:i32)
                      n338 = local read "4"() -> (w1231:i32)
                      n339 = local read "5"() -> (w1230:i32)
                      n340 = Equal?(x=w1229, y=w1234) -> (x = y?=w1239:bool)
                      n341 = Equal?(x=w1229, y=w1233) -> (x = y?=w1238:bool)
                      n342 = Equal?(x=w1229, y=w1232) -> (x = y?=w1237:bool)
                      n343 = Equal?(x=w1229, y=w1231) -> (x = y?=w1236:bool)
                      n344 = Equal?(x=w1229, y=w1230) -> (x = y?=w1235:bool)
                      n345 = Build Array(w1239, w1238, w1237, w1236, w1235) -> (w1240:bool[])
                      n346 = Or Array Elements(Boolean array=w1240) -> (logical OR=w1228:bool)
                      n347 = local write "Found Right Ball"(w1228) -> ()
                    }
                  }
                }
              }
              frame #1 {
                n348 = local read "Found Right Ball"() -> (w1247:bool)
                n349 = case shown="True" w1247 {
                  tunnel: [w1250 w1255] -> w1246
                  tunnel: w1245 -> [w1250 w1252]
                  tunnel: [w1249 w1254] -> w1244
                  tunnel: [w1248 w1253] -> w1243
                  tunnel: w1242 -> [_ w1254]
                  tunnel: w1241 -> [_ w1253]
                  frame False {
                    n350 = local read "curY"() -> (w1248:dbl)
                    n351 = local read "curX"() -> (w1249:dbl)
                  }
                  frame True {
                    n352 = Unbundle(w1252) -> ("State"=w1251:T1)
                    n353 = Bundle(cluster=w1252, "State"=w1251) -> (w1255:T9)
                  }
                }
                n354 = local write "curY"(w1243) -> ()
                n355 = local write "curX"(w1244) -> ()
              }
            }
            n356 = Unbundle By Name "Unbundle By Name"(w1170) -> ("Color classes"=w1173:i32[], "qsm.Webcam image ref"=w1159:T8)
            n357 = call "Vision Assistant5"("Image In"=w1159) -> ("Image Out"=w1157:T8, "Circles Calibrated (Shape Detection 1)"=w1158:T4, "Number of Matches (Shape Detection 1)"=w1161:i32)  [unwired: 23 in, 1 out]
            n358 = local write "Circles Calibrated (Shape Detection 1)"(w1158) -> ()
            n359 = local read "(auto) balls counter"() -> (w1174:i32)
            n360 = Bundle By Name(cluster=w1170, "qsm.Analyzed image ref"=w1157) -> (w1162:T11)
            n361 = Replace Array Subset(array=w1173, new element=w1171, index=w1174) -> (w1172:i32[])
            n362 = local read "Ready to Grab"() -> (w1166:bool)
            n363 = Bundle By Name "Bundle By Name"(cluster=w1162, "qsm.Analyzed image ref"=w1178, "Color class"=w1171, "Color classes"=w1172) -> (w1169:T11)
            n364 = case shown="True" w1166 {
              tunnel: [w1182 w1183] -> w1164
              tunnel: w1163 -> [w1181 _]
              frame False {
                n365 = Unbundle(w1181) -> ("State"=w1182:T1)
              }
              frame True {
                n366 = Unbundle(T9 {"State"=enum."Clear"} ("Shape - t, Color - f")) -> ("State"=w1183:T1)
              }
            }
            n367 = Bundle(cluster=w1163, "State"=w1164) -> (w1165:T9)
          }
          frame "(auto) Dot Controller" {
            # "here we should get and save: angle, L/R/M/G_enc's"
            # "here we should decide which of (auto) States we must use (DON'T USE 0)"
            n368 = flat-sequence {
              tunnel: w1266 -> [w1286]
              tunnel: w1265 -> [w1285]
              tunnel: w1264 -> [w1272]
              tunnel: w1263 -> [w1271]
              tunnel: w1262 -> [w1270]
              tunnel: w1261 -> [w1269]
              tunnel: [w1268] -> _
              tunnel: [w1284] -> w1260
              tunnel: w1260 -> [w1293]
              tunnel: [w1293] -> w1259
              tunnel: [w1299] -> w1258
              tunnel: w1259 -> [w1299]
              tunnel: w1257 -> [w1296]
              tunnel: [w1294] -> w1256
              frame #0 {
                n369 = local read "Angles"() -> (w1282:dbl[])
                n370 = local read "Left_enc"() -> (w1281:i32[])
                n371 = local read "Right_enc"() -> (w1280:i32[])
                n372 = local read "M_enc"() -> (w1279:i32[])
                n373 = local read "G_enc"() -> (w1278:i32[])
                n374 = Increment(x="CurDot") -> (x+1=w1283:T3)
                n375 = local write "CurDot"(w1283) -> ()
                n376 = call "(auto) SAVE.vi"("I2C Ref Out in"=w1286, "CurDot"=w1283, "Angles"=w1282, "Left_enc"=w1281, "Right_enc"=w1280, "M_enc"=w1279, "G_enc"=w1278, "error in (no error)"=w1285, "L_enc In"=w1272, "R_enc In"=w1271, "M_enc In"=w1270, "G_enc In"=w1269) -> ("I2C Ref Out out"=w1284:T23, "Angles out"=w1277:dbl[], "Left_enc out"=w1276:i32[], "Right_enc out"=w1275:i32[], "M_enc out"=w1274:i32[], "G_enc out"=w1273:i32[], "error out"=w1268:errorcluster)  [unwired: 9 in]
                n377 = local write "Angles"(w1277) -> ()
                n378 = local write "Left_enc"(w1276) -> ()
                n379 = local write "Right_enc"(w1275) -> ()
                n380 = local write "M_enc"(w1274) -> ()
                n381 = local write "G_enc"(w1273) -> ()
              }
              frame #1 {
                n382 = local read "States in total"() -> (w1292:i32)
                n383 = local read "Dots of States"() -> (w1290:i32[][])
                n384 = local read "Dots in total"() -> (w1289:i32)
                n385 = local read "CurDot"() -> (w1291:T3)
                n386 = call "(auto) Get State (SubVI).vi"("Dots in total"=w1289, "States in total"=w1292, "CurDot"=w1291, "Dots of States"=w1290) -> ("(auto) States"=w1288:T3)  [unwired: 7 in]
                n387 = local write "(auto) States"(w1288) -> ()
              }
              frame #2 {
                n388 = To Long Integer(number="(auto) States") -> (32bit integer=w1295:i32)
                n389 = Greater Than 0?(x=w1295) -> (x > 0?=w1297:bool)
                n390 = case shown="True" w1297 {
                  tunnel: w1296 -> [w1301 w1304]
                  tunnel: w1295 -> [_ w1303]
                  tunnel: [w1301 w1302] -> w1294
                  frame False {
                    n391 = local write "Stop"(TRUE ("Stop")) -> ()
                  }
                  frame True {
                    n392 = Bundle By Name(cluster=w1304, "State"=w1303) -> (w1302:T9)
                  }
                }
              }
            }
          }
          frame "(auto) Fwd (cm)" {
            n393 = call "movement forward by santimeters.vi"("error in (no error)"=w1306, "distance (cm)"=40.0) -> ("error out"=w1307:errorcluster)  [unwired: 9 in]
          }
          frame "(auto) Turn (angle)" {
            n394 = call "rotate(NORMALNOE ROTATE).vi"("On/Off\nRight/Left"=FALSE ("On/Off\nRight/Left"), "error in (no error)"=w1313) -> ("error out"=w1312:errorcluster)  [unwired: 9 in]
          }
          frame "(auto) Tnl (M2-M2.5)" {
            n395 = call "tunnel M2-M2.5.vi"("error in (no error)"=w1318) -> ("error out"=w1317:errorcluster)  [unwired: 10 in]
          }
          frame "Wait for button" {
            n396 = while {
              stop <- w1329 stop-if-true
              n397 = local read "Stop"() -> (w1331:bool)
              n398 = xnode "Button 2"() -> ("Value"=w1327:bool)  [unwired: 1 in, 1 out]
              n399 = Or(x="Next step", y=w1331) -> (x .or. y?=w1328:bool)
              n400 = Or(x=w1328, y=w1327) -> (x .or. y?=w1329:bool)
            }
            n401 = local write "Next step"(FALSE ("Look at ball")) -> ()
          }
        }
        n402 = xnode "Digital output (1 sample)"("Left+ (A/DIO5 (Pin 21))"="Left+", "Right+ (A/DIO7 (Pin 25))"="Right+", "Left- (A/DIO6 (Pin 23))"="Left-", "Right- (A/DIO13 (Pin 26))"="Right-", "error in (no error)"=w134) -> ("error out"=w184:errorcluster)
        n403 = xnode "Digital output (1 sample) 2"("G- (B/DIO7 (Pin 25))"="G-", "G+ (B/DIO13 (Pin 26))"="G+", "M+ (B/DIO5 (Pin 21))"="M+", "M- (B/DIO6 (Pin 23))"="M-", "error in (no error)"=w125) -> ("error out"=w183:errorcluster)
        n404 = Merge Errors(w184, w183) -> (w172:errorcluster)
        n405 = local read "ball match"() -> (w147:bool)
        n406 = local read "pattern match"() -> (w145:bool)
        n407 = Or(x=w147, y="ball = pattern?") -> (x .or. y?=w148:bool)
        n408 = Or(x=w148, y=w145) -> (x .or. y?=w146:bool)
        n409 = xnode "LED"("LED0"=w146, "LED1"=w146, "LED2"=w146, "LED3"=w146, "error in (no error)"=w172) -> ("error out"=w171:errorcluster)
        n410 = Unbundle(w97) -> ("State"=→"CurState":T1)
        n411 = Unbundle By Name(w95) -> ("Pattern classes"=w170:i32[], "Color classes"=w163:i32[])
        "Color classes" <- w163
        "Pattern classes" <- w170
        n412 = Merge Errors(w164, w171) -> (w186:errorcluster)
        n413 = local read "Number of Matches (Shape Detection 1)"() -> (w169:i32)
        n414 = local read "Ball number"() -> (w162:i32)
        n415 = Index Array(array=w170) -> (element=w149:i32)  [unwired: 1 in]
        n416 = Index Array(array=w163, index=w162) -> (element=w150:i32)
        n417 = Equal?(x=w150, y="1") -> (x = y?=→"1b":bool)
        n418 = Equal?(x=w150, y="2") -> (x = y?=→"2b":bool)
        n419 = Equal?(x=w150, y="3") -> (x = y?=→"3b":bool)
        n420 = Equal?(x=w150, y="4") -> (x = y?=→"4b":bool)
        n421 = Equal?(x=w150, y="5") -> (x = y?=→"5b":bool)
        n422 = Equal?(x=w149, y=w150) -> (x = y?=w165:bool)
        n423 = local write "ball = pattern?"(w165) -> ()
        n424 = Greater Than 0?(x=w169) -> (x > 0?=w168:bool)
        n425 = case shown="True" w168 {
          tunnel: [w232 w238] -> w167
          tunnel: w95 -> [w231 w238]
          frame False {
            n426 = Unbundle By Name(w231) -> ("Color classes"=w228:i32[])
            n427 = for {
              N: 5 -> [w236]
              tunnel: [w237] -> w230
              tunnel: w228 -> [w234]
              n428 = Decrement(x=w236) -> (x-1=w235:i32)
              n429 = Replace Array Subset(array=w234, new element=20, index=w235) -> (w237:i32[])
            }
            n430 = Bundle By Name(cluster=w231, "Color classes"=w230) -> (w232:T11)
          }
          frame True {
          }
        }
      }
    }
    frame #1 {
      w1367 = 0 ("(auto) balls counter")
      w1380 = 0 ("G_upper bound")
      w1390 = 1 ("Ball index")
      w1368 = FALSE ("X is in range")
      n431 = disable-structure shown="Disabled" {
        disable-tunnel: w1386 -> [w1394 _]
        disable-tunnel: [w1393 _] -> w1385
        disable-tunnel: w1381 -> [w1392 _]
        frame Disabled {
          n432 = call <vilib>:"Close.vi"("error in (no error)"=w1392, "I2C Ref In"=w1394) -> ("error out"=w1393:errorcluster)  [unwired: 9 in]
        }
        frame Enabled {
        }
      }
      n433 = call "Setup manipulator (SubVI).vi"("Reverse?"=TRUE ("Release?"), "G_upper bound"=w1380, "M_lower bound"=w1380, "error in (no error)"=w1381, "M_Encoder Ref In"=w1377, "G_Encoder Ref In"=w1376) -> ("error out"=w1374:errorcluster)  [unwired: 9 in]
      n434 = call <vilib>:"Close.vi"("error in (no error)"=w1381, "PWM Ref In"=w1379) -> ("error out"=w1387:errorcluster)  [unwired: 9 in]
      n435 = call <vilib>:"Close.vi"("error in (no error)"=w1381, "PWM Ref In"=w1378) -> ("error out"=w1388:errorcluster)  [unwired: 9 in]
      n436 = call <vilib>:"Close.vi"("error in (no error)"=w1374, "Encoder Ref In"=w1377) -> ("error out"=w1382:errorcluster)  [unwired: 9 in]
      n437 = call <vilib>:"Close.vi"("error in (no error)"=w1374, "Encoder Ref In"=w1376) -> ("error out"=w1383:errorcluster)  [unwired: 9 in]
      n438 = call <vilib>:"Close.vi"("error in (no error)"=w1374, "Encoder Ref In"=w1372) -> ("error out"=w1371:errorcluster)  [unwired: 9 in]
      n439 = call <vilib>:"Close.vi"("error in (no error)"=w1374, "Encoder Ref In"=w1373) -> ("error out"=w1370:errorcluster)  [unwired: 9 in]
      n440 = Merge Errors(w1385, w1381, w1387, w1388, w1382, w1383, w1371, w1370) -> (w1389:errorcluster)
      n441 = local write "(auto) balls counter"(w1367) -> ()
      n442 = local write "Ball number"(w1390) -> ()
      n443 = local write "pattern number"(w1390) -> ()
      n444 = call <vilib>:"Simple Error Handler.vi"("error in (no error)"=w1389) -> ("error out"=w1391:errorcluster)  [unwired: 4 in, 4 out]
      "error out" <- w1391
      n445 = local write "curY"(w1367) -> ()
      n446 = local write "curX"(w1367) -> ()
      n447 = local write "ball = pattern?"(w1368) -> ()
      n448 = local write "X is in range"(w1368) -> ()
      n449 = local write "R_PWM"("Def PWM") -> ()
      n450 = local write "Y is in range"(w1368) -> ()
      n451 = local write "L_PWM"("Def PWM") -> ()
      n452 = local write "Next step"(w1368) -> ()
      n453 = shared-variable "myRIO-1900\\vars.lvlib\\def Z"(ext -800.0 ("def Z")) -> ()  [unwired: 1 in, 1 out]
      n454 = local write "Ready to Grab"(w1368) -> ()
      n455 = local write "Right+"(w1368) -> ()
      n456 = local write "Right-"(w1368) -> ()
      n457 = local write "rotate"(w1368) -> ()
      n458 = local write "Left+"(w1368) -> ()
      n459 = local write "Left-"(w1368) -> ()
      n460 = local write "Stop"(w1368) -> ()
      n461 = local write "M+"(w1368) -> ()
      n462 = local write "G+"(w1368) -> ()
      n463 = local write "M-"(w1368) -> ()
      n464 = local write "G-"(w1368) -> ()
    }
  }
  n465 = call <vilib>:"Reset myRIO.vi"("error in (no error)"=w52) -> ()  [unwired: 10 in, 1 out]
